vi "HMF_Factorial.vi"() -> ()   [LabVIEW 2015]
uses:
  <vilib>/Platform/TimedLoop/XDataNode/timing_clust.ctl
  <vilib>/Platform/TimedLoop/XDataNode/nitl_modes.ctl
  <vilib>/Platform/TimedLoop/XDataNode/wakeup.ctl
  <vilib>/DAQmx/read.llb/DAQmx Read (Analog DBL 1Chan 1Samp).vi
  <vilib>/DAQmx/read.llb/DAQmx Read (Analog 1D DBL NChan 1Samp).vi
  <vilib>/DAQmx/create/channels.llb/DAQmx Create Channel (AI-Voltage-Basic).vi
  <vilib>/Enthought/Python Integration Toolkit/api/Unpack Double.vi
  <vilib>/DAQmx/miscellaneous.llb/DAQmx Fill In Error Info.vi
  <vilib>/Platform/TimedLoop/XDataNode/XDataNode.xnode
  Program Files/neMESYS_SDK/neMESYS LabVIEW Kit/neMESYS LabVIEW Integration Kit.lvlib
  <vilib>/Platform/TimedLoop/XDataNode/XDNodeRunTimeDep.lvlib
  Conor/Temp CN7500/Omega CN7500/Omega CN7500.lvlib
  <vilib>/Enthought/Python Integration Toolkit/Python Integration Toolkit.lvlib
panel:
  in  "Temp  Limit OFF or ON":bool
  out "syringe limit empty":bool
  out "Pressure limit reached":bool
  out "Temp limit reached":bool
  in  "NaOH in 3 or NaOH in 2":bool
  out "N2 Cal 4":dbl
  out "N2 Cal 3":dbl
  out "N2 Cal 2":dbl
  out "O2 Cal 1":dbl
  out "C FDCA 8":dbl
  out "C FFCA 8":dbl
  out "C FDCA 7":dbl
  out "C FFCA 7":dbl
  out "C FDCA 6":dbl
  out "C FFCA 6":dbl
  out "C FDCA 5":dbl
  out "C FFCA 5":dbl
  out "C FDCA 4":dbl
  out "C FFCA 4":dbl
  out "C FDCA 3":dbl
  out "C FFCA 3":dbl
  out "C FDCA 2":dbl
  out "C FFCA 2":dbl
  out "C FDCA 1":dbl
  out "C FFCA 1":dbl
  out "O2 frac 8":dbl
  in  "O2 frac 8":dbl
  out "O2 frac 7":dbl
  in  "O2 frac 7":dbl
  out "O2 frac 6":dbl
  in  "O2 frac 6":dbl
  out "O2 frac 5":dbl
  in  "O2 frac 5":dbl
  out "O2 frac 4":dbl
  in  "O2 frac 4":dbl
  out "O2 frac 3":dbl
  in  "O2 frac3":dbl
  out "O2 frac 2":dbl
  out "O2 frac 1":dbl
  in  "O2 frac 2":dbl
  in  "O2 frac 1":dbl
  in  "O2 frac 0":dbl
  in  "Total Gas Flow Rate":dbl
  in  "Back Pressure Bar Abs":dbl
  in  "Test Gas Communication":bool
  in  "Read Set Points":bool
  in  "Change New Set Points":bool
  out "Text Read From Clipboard 5":string
  out "Read error out 5":errorcluster
  out "Write Set Point Status 2":string
  out "Error Out 5":i32
  out "Write error out 5":errorcluster
  out "Text Read From Clipboard 4":string
  out "Read error out 4":errorcluster
  out "Write Set Point Status":string
  out "Error Out 4":i32
  out "Write error out 4":errorcluster
  in  "Set Point 1 (NmL/min)":dbl
  in  "Set Point 2 (NmL/min)":dbl
  in  "Set Point 3 (NmL/min)":dbl
  out "Flow Span of All Controlers (NmL/min)":dbl
  in  "Set Point 4 (NmL/min)":dbl
  out "Set Point Function":string
  out "Text Read From Clipboard 3":string
  out "Read error out 3":errorcluster
  out "Read Set Point Status":string
  out "Error Out 3":i32
  out "Write error out 3":errorcluster
  out "Text Read From Clipboard":string
  out "Read error out":errorcluster
  out "Test Status":string
  out "Error Out":i32
  out "Write error out":errorcluster
  out "Text Read From Clipboard 2":string
  out "Read error out 2":errorcluster
  out "Read Flow Status":string
  out "Gas Flow 1 NmL/min":dbl
  out "Gas Flow 2 NmL/min":dbl
  out "Gas Flow 3 NmL/min":dbl
  out "Gas Flow 4 NmL/min":dbl
  out "Gas Flow rate":dynamicdata(graph)
  out "First waste string":string
  out "Rest of string 1":string
  out "First Number":string
  out "Rest of string 2":string
  out "Second Number 2":string
  out "Rest of string 3":string
  out "Third Number 3":string
  out "Rest of string 4":string
  out "Fourth Number 3":string
  out "Rest of string 5":string
  out "Error Out 2":i32
  out "Write error out 2":errorcluster
  out "Nitrogen Pressure (barg)":dbl
  out "Reactor Gas Back Pressure (barg)":dbl
  out "Nitrogen Gas  Pressure (barg)":dbl
  out "Slope 4":dbl
  out "Slope 3":dbl
  out "Slope 2":dbl
  out "Intercept 4":dbl
  out "Intercept  3":dbl
  out "Intercept 2":dbl
  out "Intercept 1":dbl
  out "Slope 1":dbl
  in  "2 Syringes or 4 Syringes":bool
  in  "Conc NaOH in Syringe":dbl
  in  "Cat Mass mg":dbl
  out "Exp 2":bool
  out "C HFCA 1":dbl
  out "C HMF 1":dbl
  out "Exp 9":bool
  out "Liquid Inlet Pressure (bar g)":dbl
  in  "Liquid P sensor Terminal Configuration":i32(ring)=-1 items=["default"=-1, "RSE"=10083, "NRSE"=10078, "Differential"=10106, "Pseudodifferential"=12529]
  in  "Liquid P sensor Physical Channel":tag="Dev1/ai0"
  in  "Temp 2":dbl
  in  "Conc 2":dbl
  in  "Flow 2":dbl
  out "Exp 8":bool
  out "Exp 7":bool
  out "Exp 6":bool
  out "Exp 5":bool
  out "Exp 4":bool
  out "Exp 3":bool
  out "Exp 1":bool
  out "Exp 0":bool
  out "C HMF 8":dbl
  out "C HFCA 8":dbl
  in  "Flow 8":dbl
  in  "Conc 8":dbl
  in  "Temp 8":dbl
  out "Temp 8":dbl
  out "Flow 8":dbl
  out "Conc 8":dbl
  out "C HMF 7":dbl
  out "C HFCA 7":dbl
  in  "Flow 7":dbl
  in  "Conc 7":dbl
  in  "Temp 7":dbl
  out "Temp 7":dbl
  out "Flow 7":dbl
  out "Conc 7":dbl
  out "C HMF 6":dbl
  out "C HFCA 6":dbl
  in  "Flow 6":dbl
  in  "Conc 6":dbl
  in  "Temp 6":dbl
  out "Temp 6":dbl
  out "Flow 6":dbl
  out "Conc 6":dbl
  out "C HMF 5":dbl
  out "C HFCA 5":dbl
  in  "Flow 5":dbl
  in  "Conc 5":dbl
  in  "Temp 5":dbl
  out "Temp 5":dbl
  out "Flow 5":dbl
  out "Conc 5":dbl
  out "C HMF 4":dbl
  out "C HFCA 4":dbl
  out "Conc 1":dbl
  out "Flow 1":dbl
  out "Temp 1":dbl
  out "Conc 2":dbl
  out "Flow 2":dbl
  out "Temp 2":dbl
  in  "Flow 4":dbl
  in  "Conc 4":dbl
  in  "Temp 4":dbl
  out "Temp 4":dbl
  out "Flow 4":dbl
  out "Conc 4":dbl
  out "C HMF 3":dbl
  out "C HFCA 3":dbl
  out "Conc 3":dbl
  out "Flow 3":dbl
  out "Temp 3":dbl
  out "C HMF 2":dbl
  out "C HFCA 2":dbl
  in  "Temp 3":dbl
  in  "Conc 3":dbl
  in  "Flow 3":dbl
  in  "Result file name -  needs extension RecordHMF.xlsx":string
  in  "HPLC file Name -doesnt need extension":string
  out "Desired Conc Not Possible":bool
  in  "Safety or Emergency Syringe Control":bool
  out "Feed Concentration if 2 syringe (M)":dbl
  out "Total Flowrate (uL/min)":dbl
  out "Oxygen Gas Pressure (barg)":dbl
  in  "Shut down in empty?\nLeft off, right on":bool
  out "Safety Shut Down Pressure (barg)":dbl
  out "Safety Shut Down Temp":dbl
  out "Actual Temp (oC)":dbl
  out "Temperature":dynamicdata(graph)
  out "Temp Set Point (oC)":dbl
  in  "Temp 1":dbl
  in  "Temp 0":dbl
  in  "Update Temperature Set Point":bool
  in  "Automated Experiments or Direct Control":bool
  in  "Set Point (oC)":dbl
  out "loop ind":dbl
  in  "Stop everything":bool
  in  "Skip Exp":bool
  in  "Minutes between Exp":dbl min=0.0 step=0.05
  in  "Refill 4":bool
  in  "Refill 3":bool
  in  "Refill 2":bool
  in  "Refill 1":bool
  in  "Empty 4":bool
  in  "Empty 3":bool
  in  "Empty 2":bool
  in  "Empty 1":bool
  in  "Calibrate 4":bool
  in  "Calibrate 3":bool
  in  "Calibrate 2":bool
  in  "Calibrate 1":bool
  in  "Stop Dose 4":bool
  in  "Stop Dose 3":bool
  in  "Stop Dose 2":bool
  in  "Stop Dose 1":bool
  in  "Flow 1":dbl
  in  "Conc 1":dbl
  in  "Flow 0":dbl
  in  "Conc 0  (M)":dbl
  in  "Generate Flow":bool
  in  "Set Flowrate 1":dbl
  in  "Set Flowrate 2":dbl
  in  "Set Flowrate 3":dbl
  in  "Set Flowrate 4":dbl
  out "High Conc":dbl min=0.0 max=2.0
  out "Low Conc":dbl min=0.0 max=2.0
  out "Syringe Level 4":dbl(slide) scale=0.0..5500.0
  out "Syringe Level 3":dbl(slide) scale=0.0..5500.0
  out "Syringe Level 2":dbl(slide) scale=0.0..5500.0
  out "Syringe Level 1":dbl(slide) scale=0.0..5500.0
  out "Flowrate 4 NaOH":dbl
  out "Flowrate 3 NaOH":dbl
  out "Flowrate 2 NaOH or HMF":dbl
  out "Flowrate 1 HMF":dbl
  # "Current Conditions"
  # "Pre Planned Experiments"
  # "Conducted Experiments Set Points"
  # "example file name to show correct format is..."
  # "HMF_HPLC"
  # "(uL/min)"
  # "Coerced to nearest possible"
  # "Factorial Only"
  # "Experimental Info"
  # "Direct Control"
  # "Emergency Syringe Control Below"
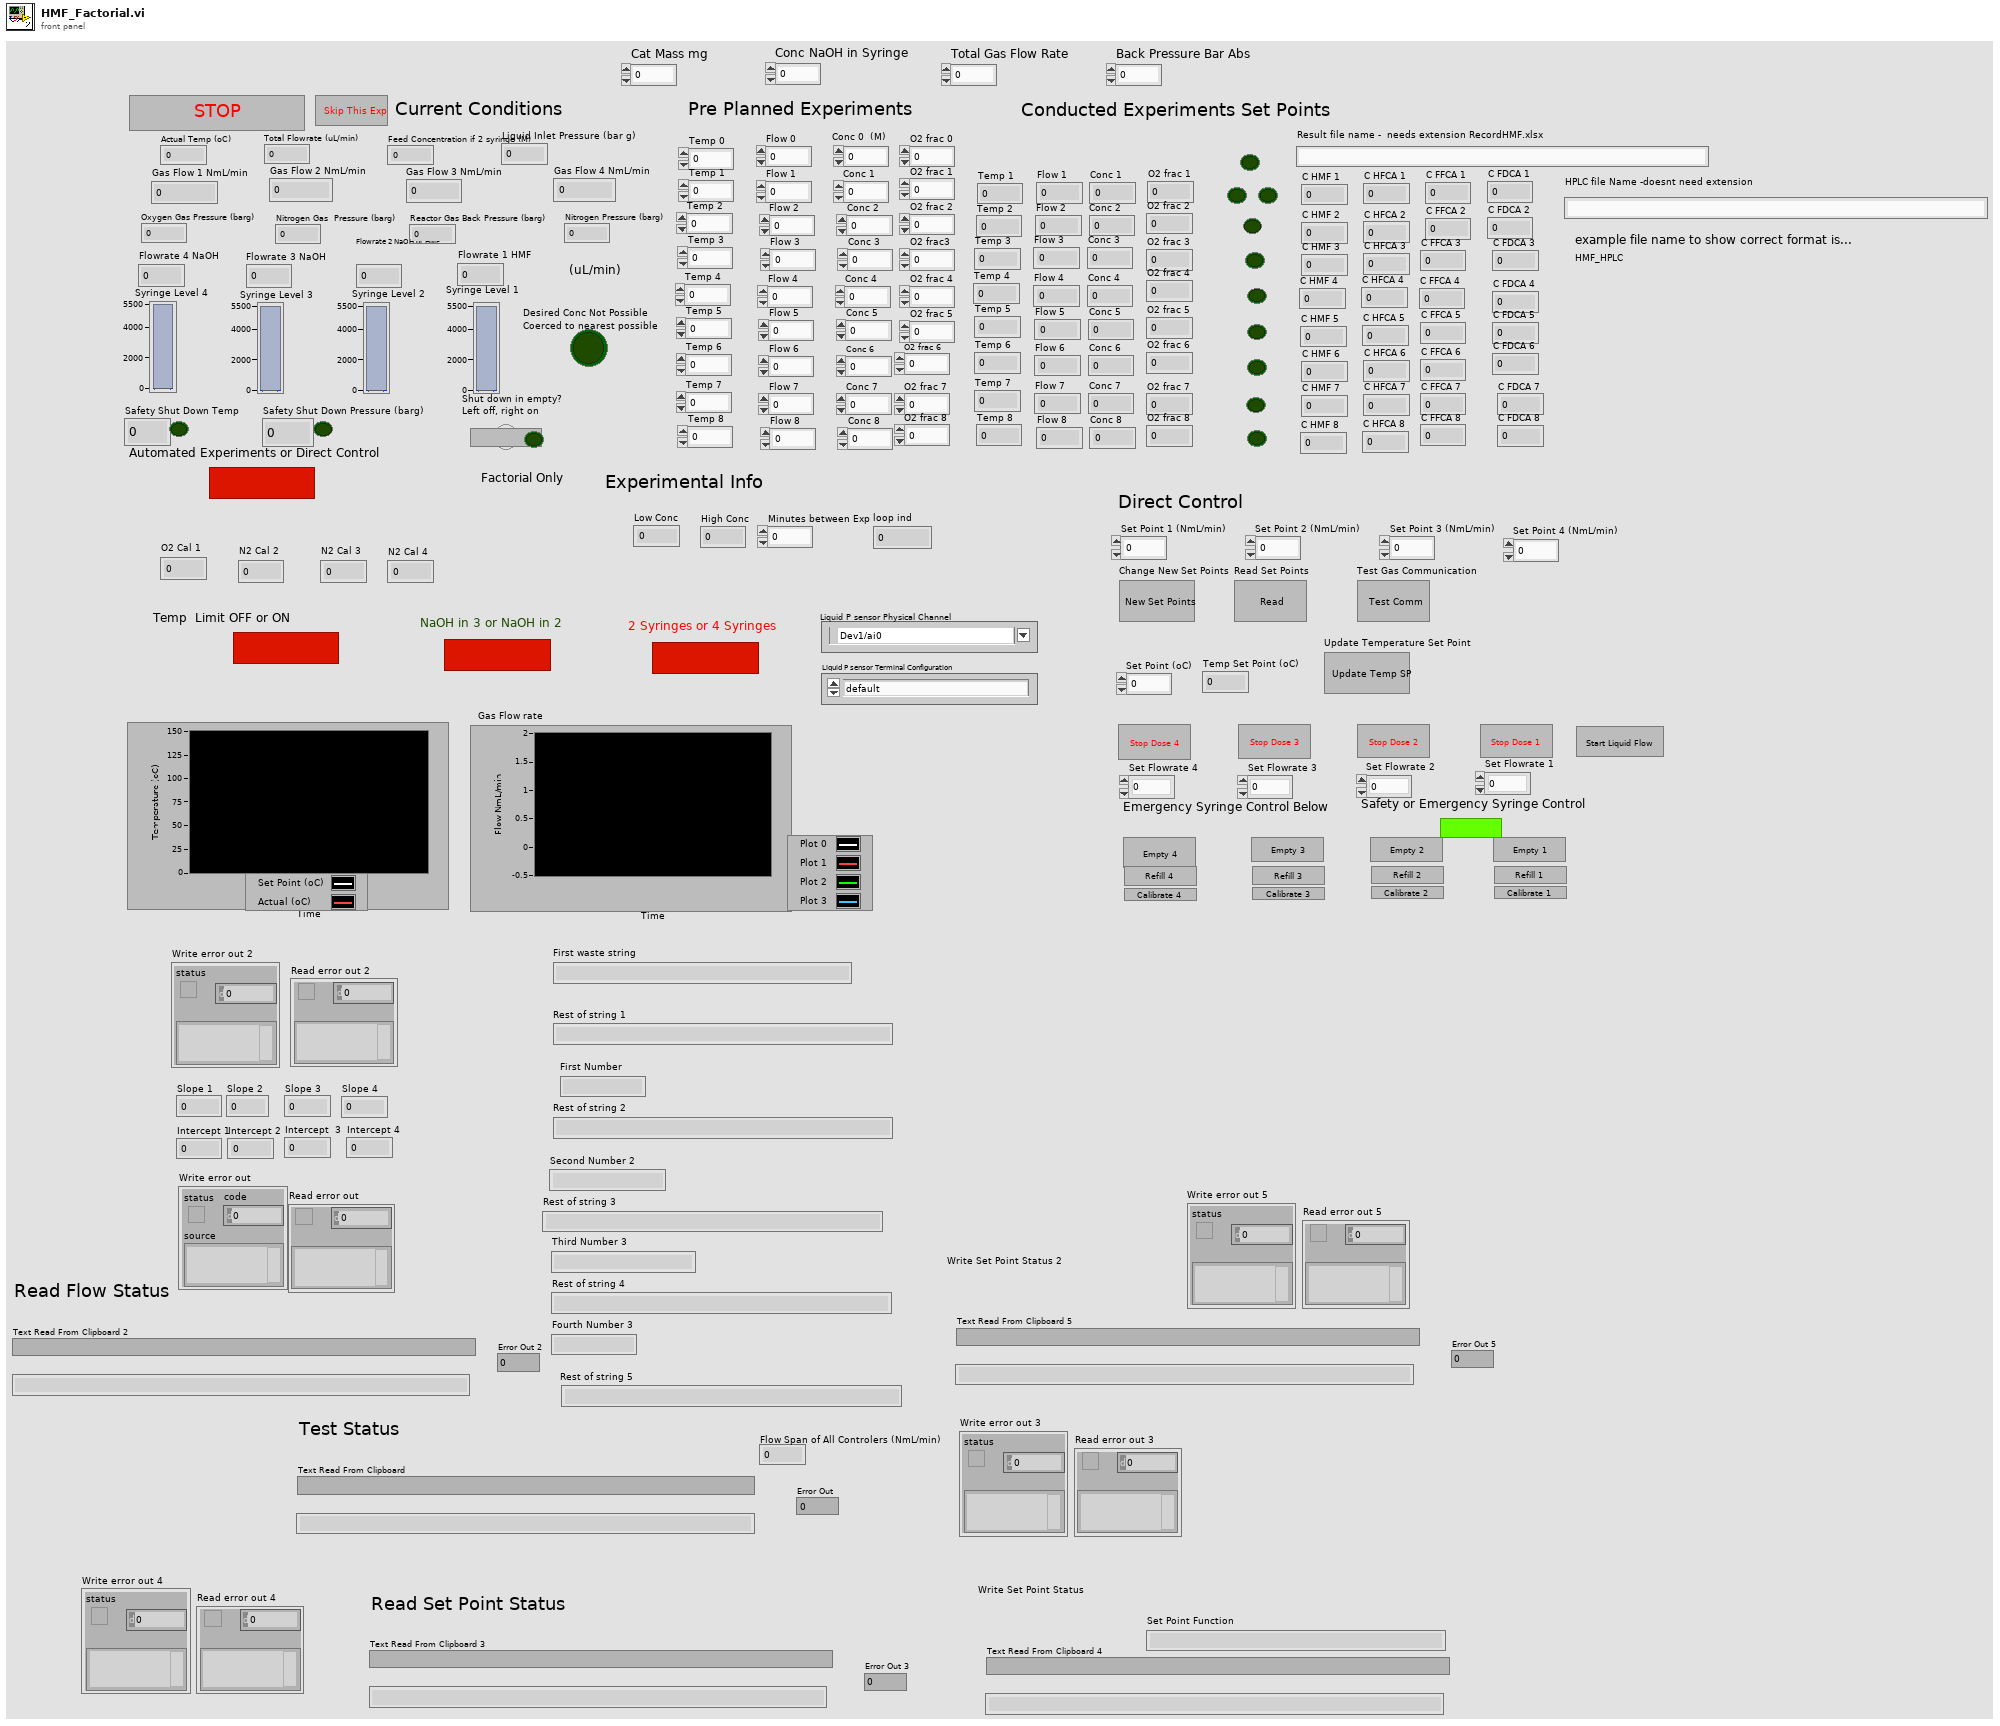
[diagram p1: front panel]
types:
  T1 = typedef "XDNodeRunTimeDep.lvlib/timing_clust.ctl" = cluster{"Expected End [f-1]":u64, "Actual End [f-1]":u64, "Finished Late? [f-1]":bool, "Expected End [i-1]":u64, "Actual End [i-1]":u64, "Finished Late? [i-1]":bool, "Expected Start [i]":u64, "Actual Start [i]":u64, "Expected Start [f]":u64, "Actual Start [f]":u64, "Source Name":string, "Structure Name":string, "Period":i64, "Deadline":i64, "Offset":i64, "Start":i64, "Priority":i32, "Timeout":i32, "Mode":T2, "Wakeup Reason":T3, "Error":errorcluster, "Source Type":string, "Secondary Source Type":string, "Global End Time":u64, "Global Start Time":u64, "Frame Duration":u64, "Iteration Duration":u64, "Assigned CPU":i32, "I/O Scan Engine Mode":u32}
  T2 = typedef "XDNodeRunTimeDep.lvlib/nitl_modes.ctl" = enum32{"No Change", "Process missed periods, maintain original phase", "Discard missed periods, maintain original phase", "Process missed periods, ignore original phase", "Discard missed periods, ignore original phase"}
  T3 = typedef "XDNodeRunTimeDep.lvlib/wakeup.ctl" = enum32{"Normal", "Aborted", "Asynchronous wakeup", "Timing source error", "Timed loop error", "Timeout"}
  T4 = typedef "Python Integration Toolkit.lvlib/Session ID.ctl" = u64
  T5 = typedef "Python Integration Toolkit.lvlib/Python Objects.ctl" = variant
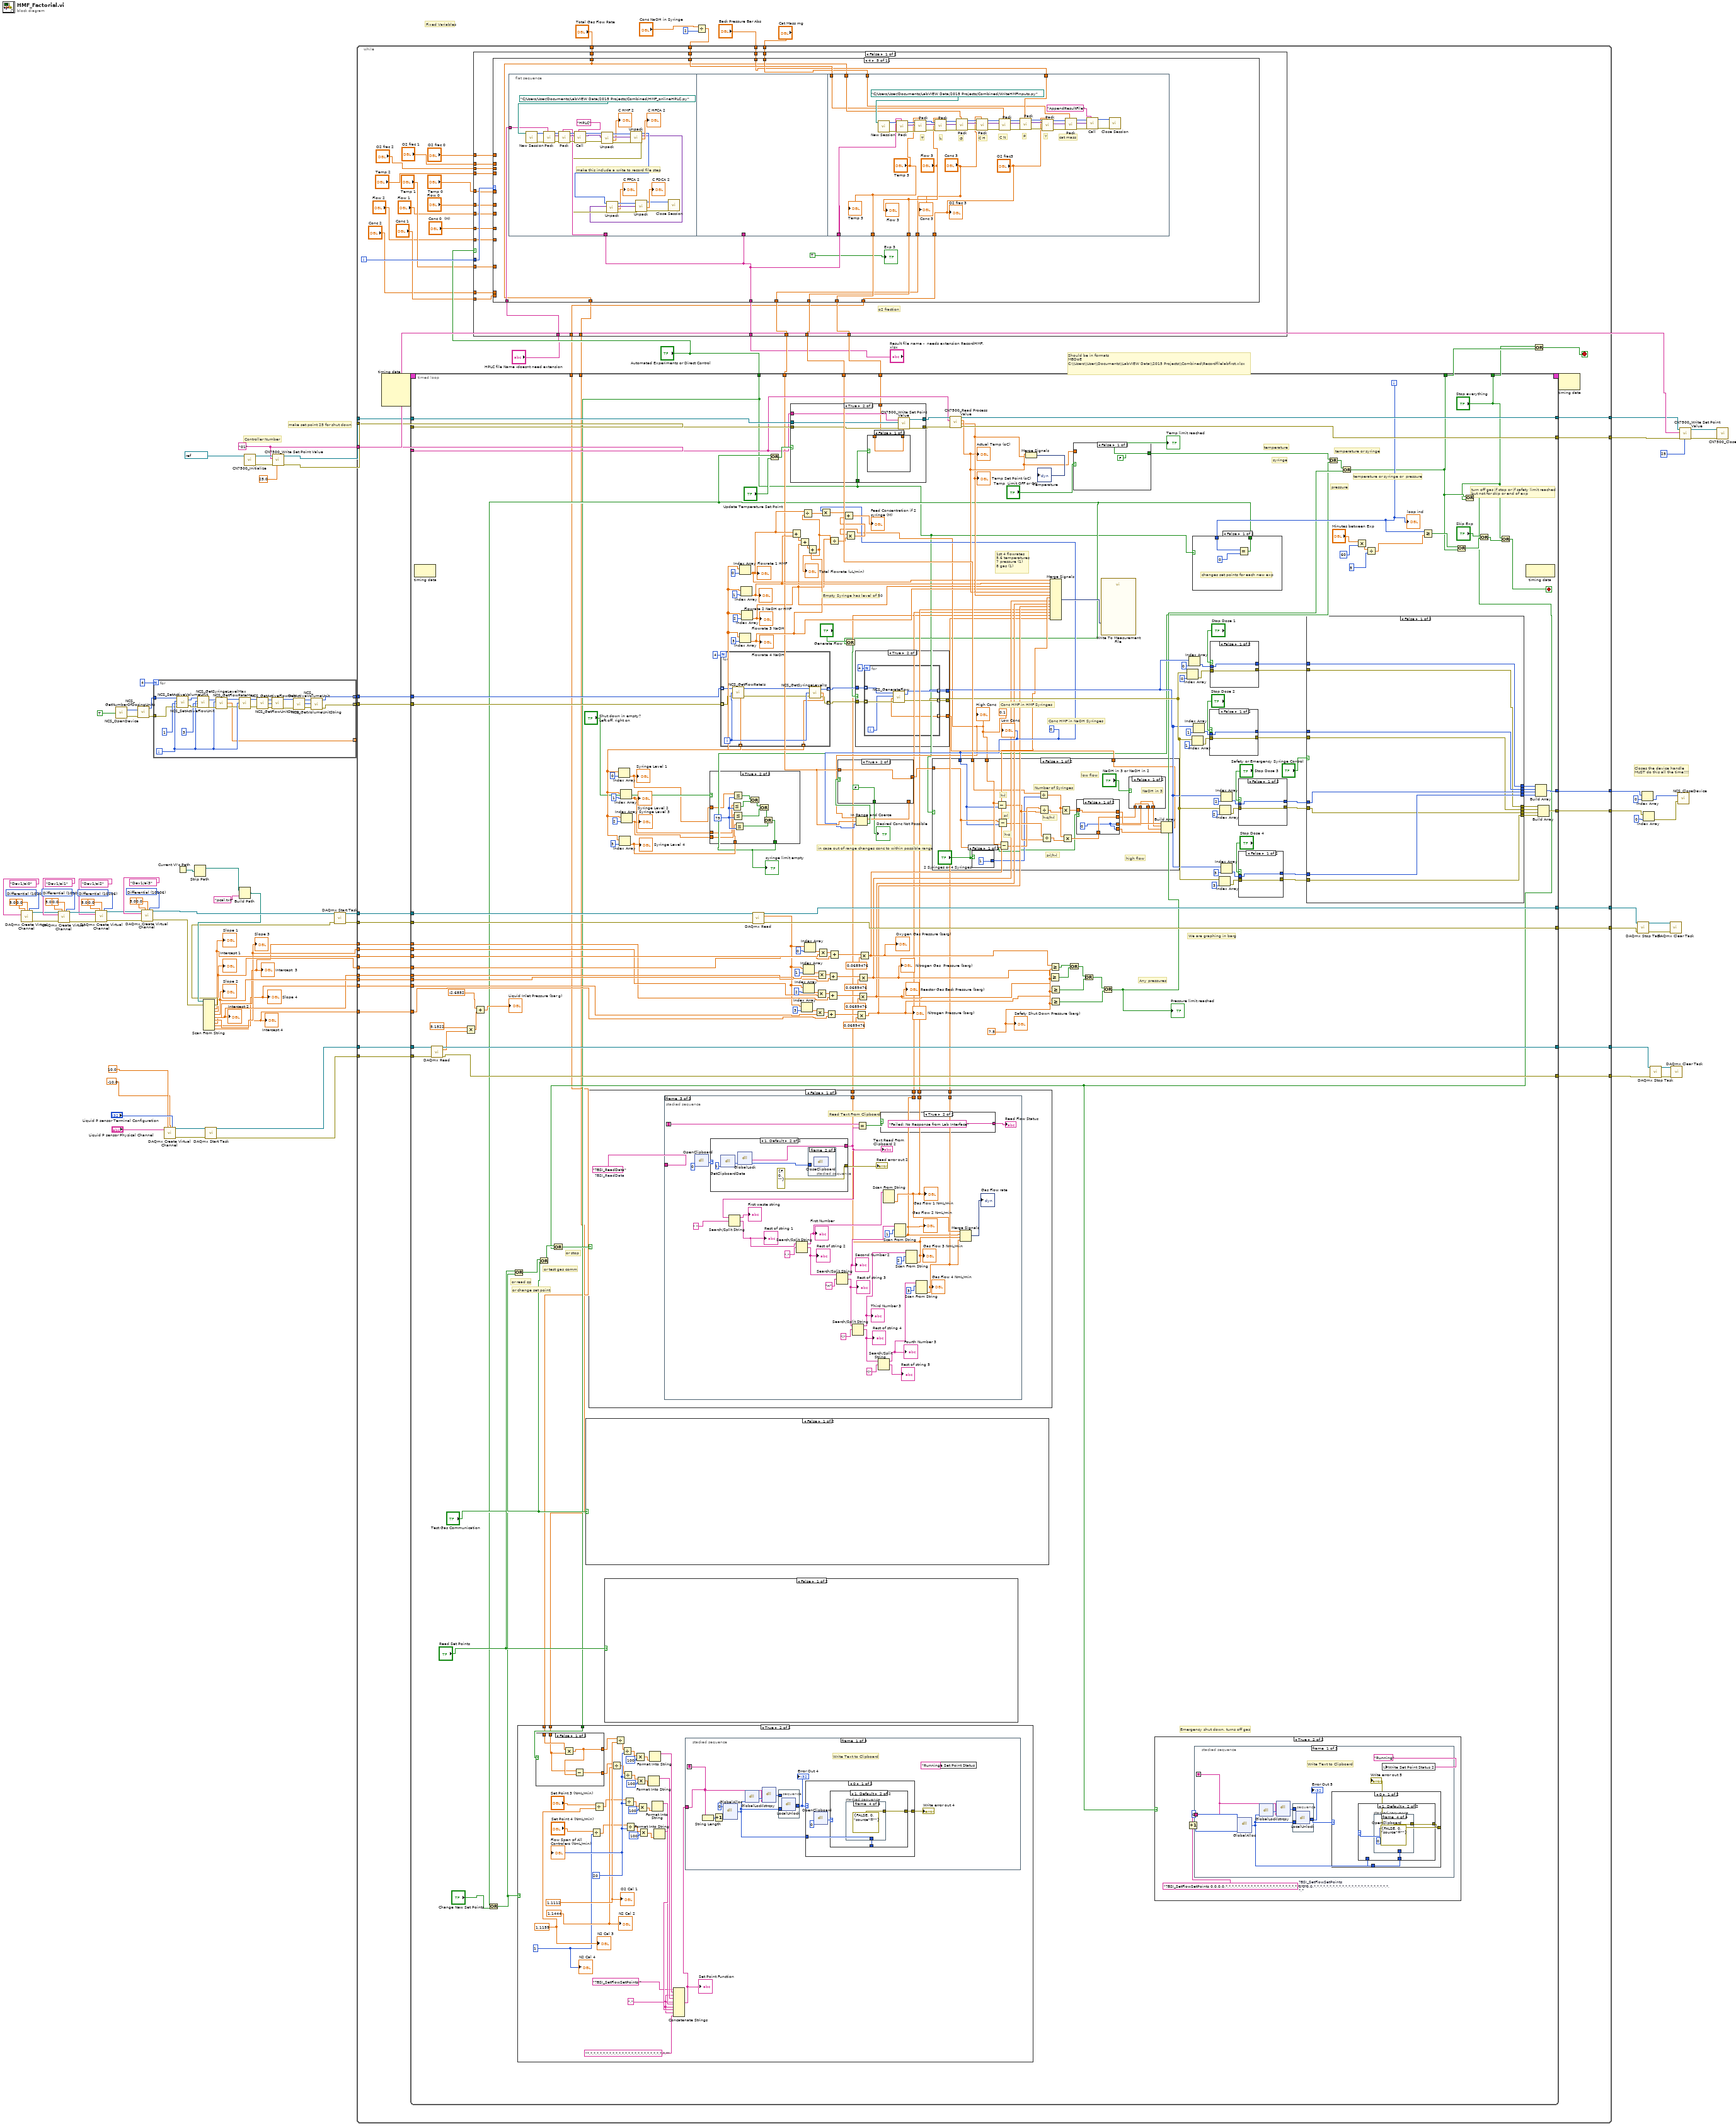
[diagram p0: block diagram]
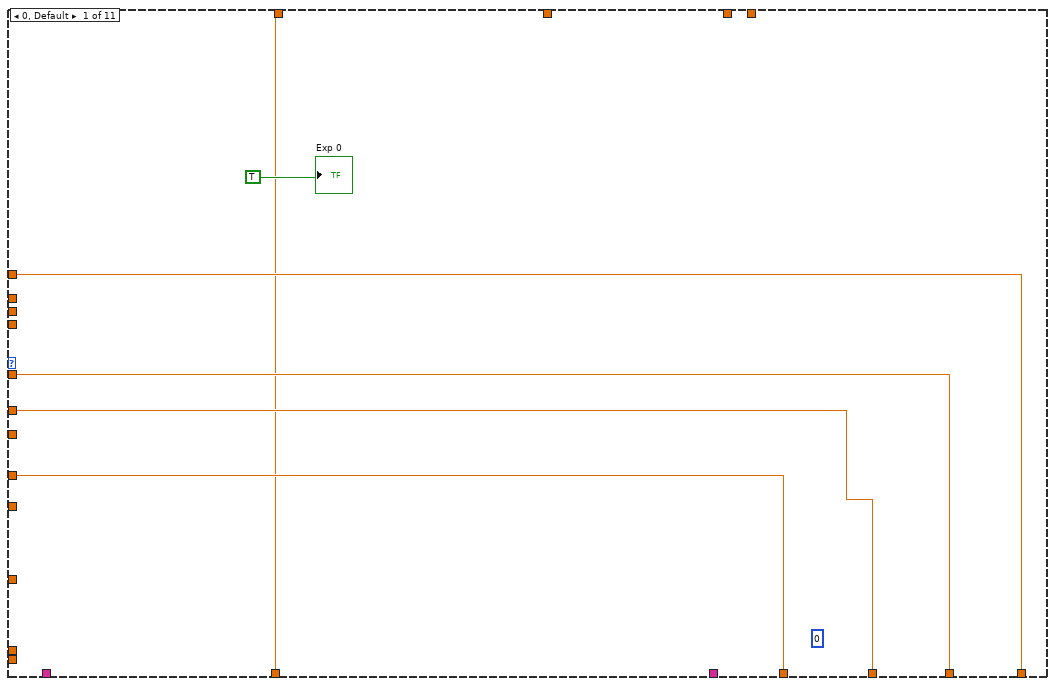
[diagram p2: hidden frame]
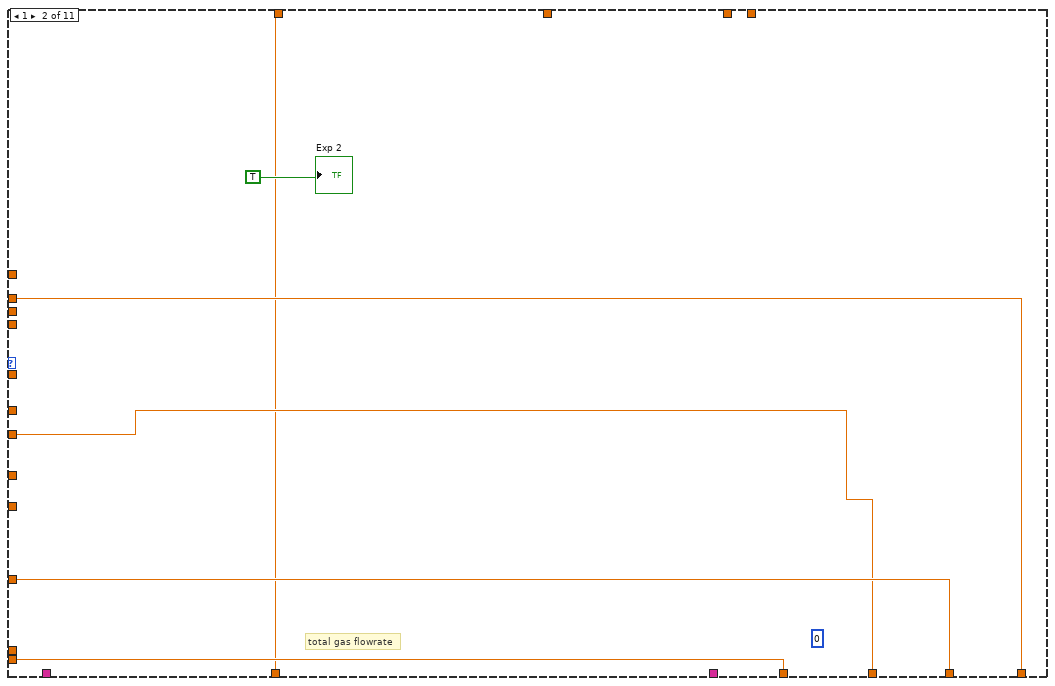
[diagram p3: hidden frame]
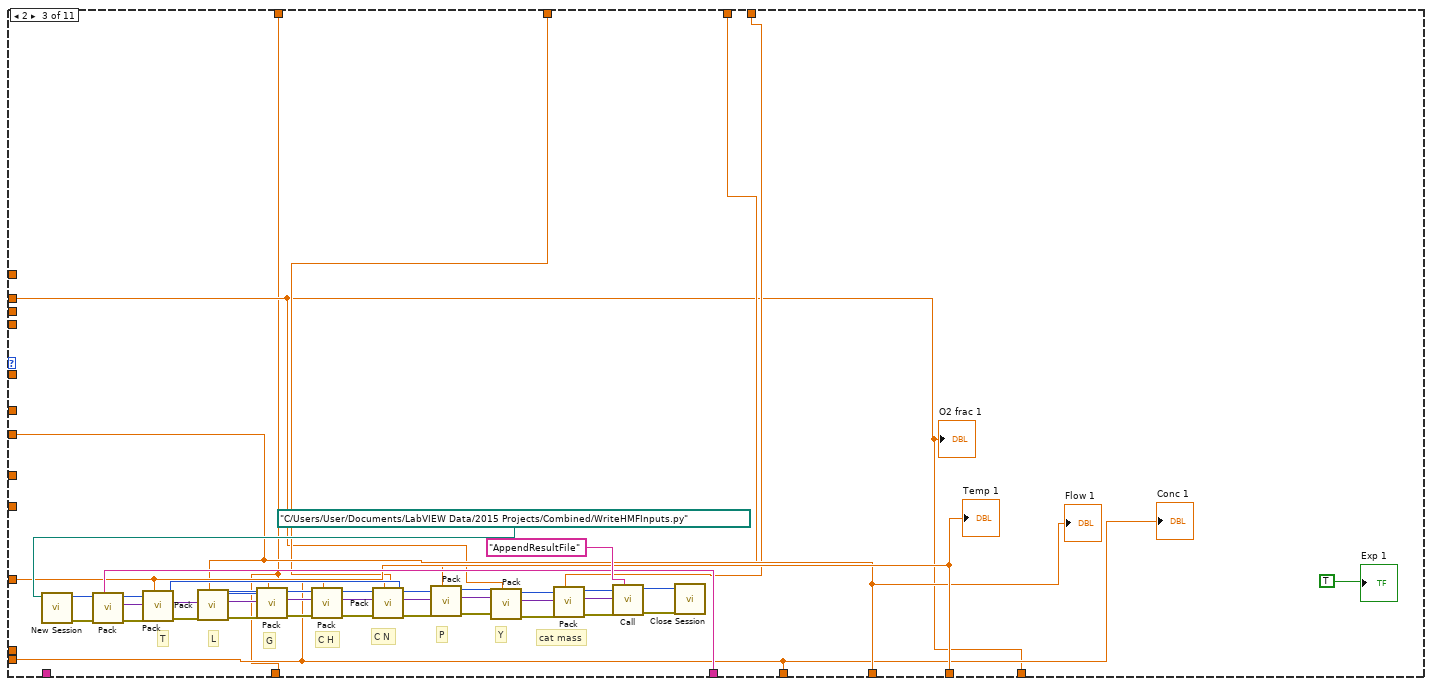
[diagram p4: hidden frame]
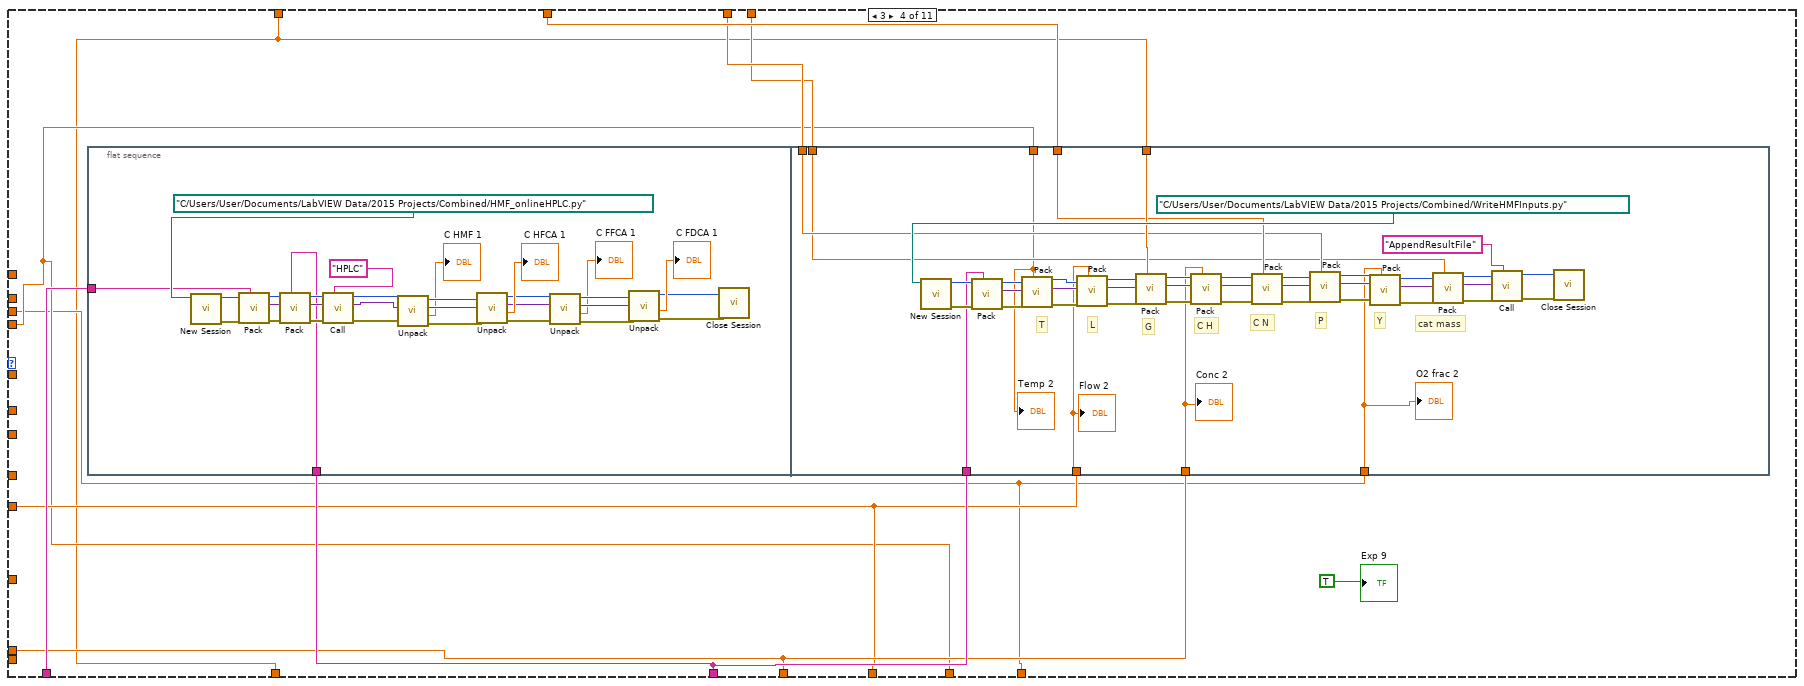
[diagram p5: hidden frame]
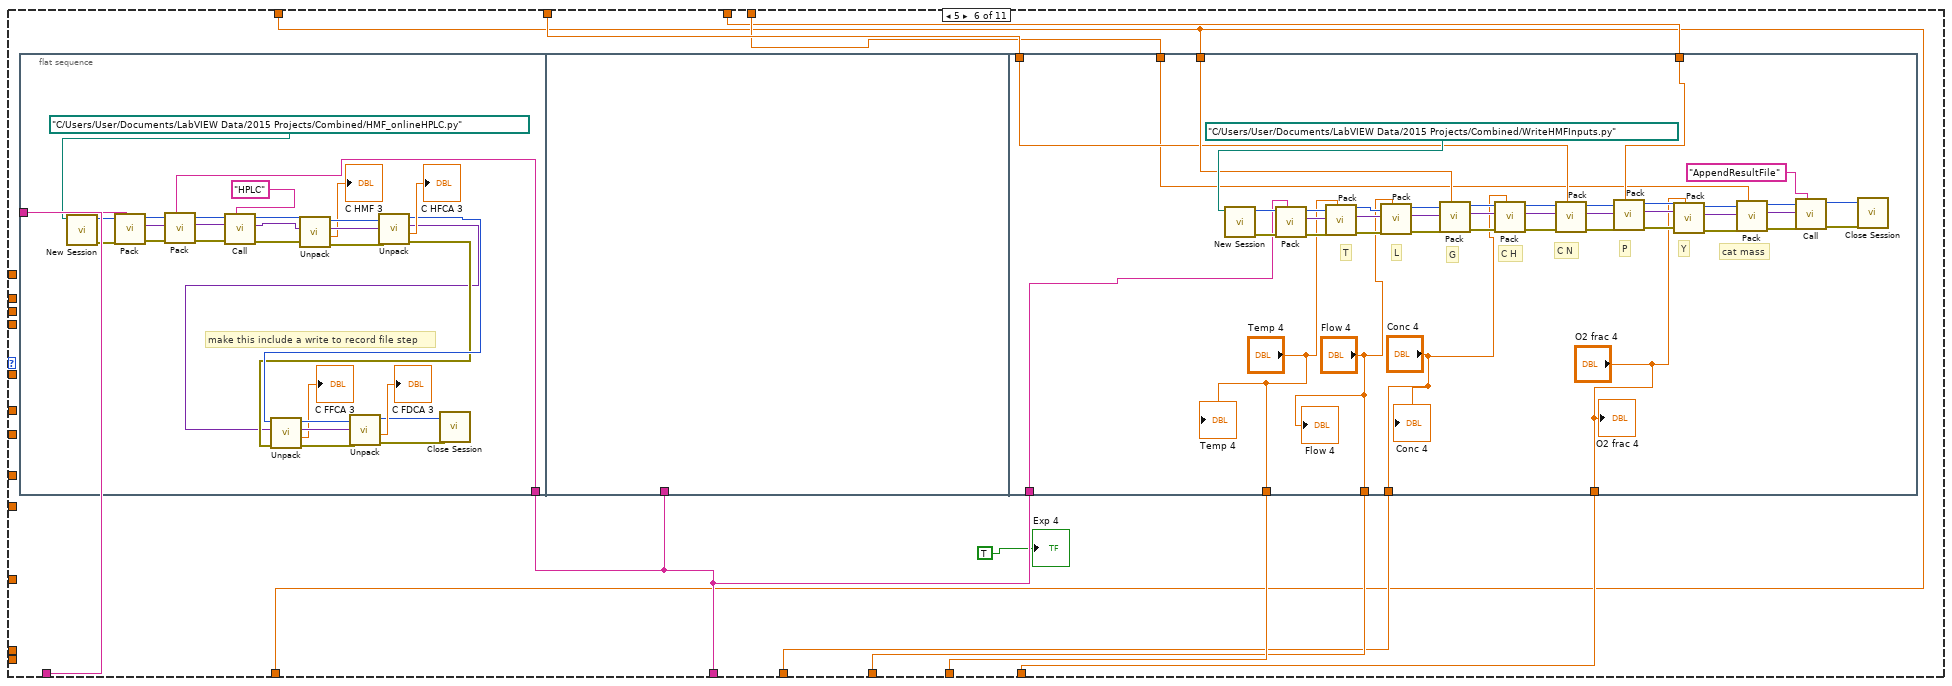
[diagram p6: hidden frame]
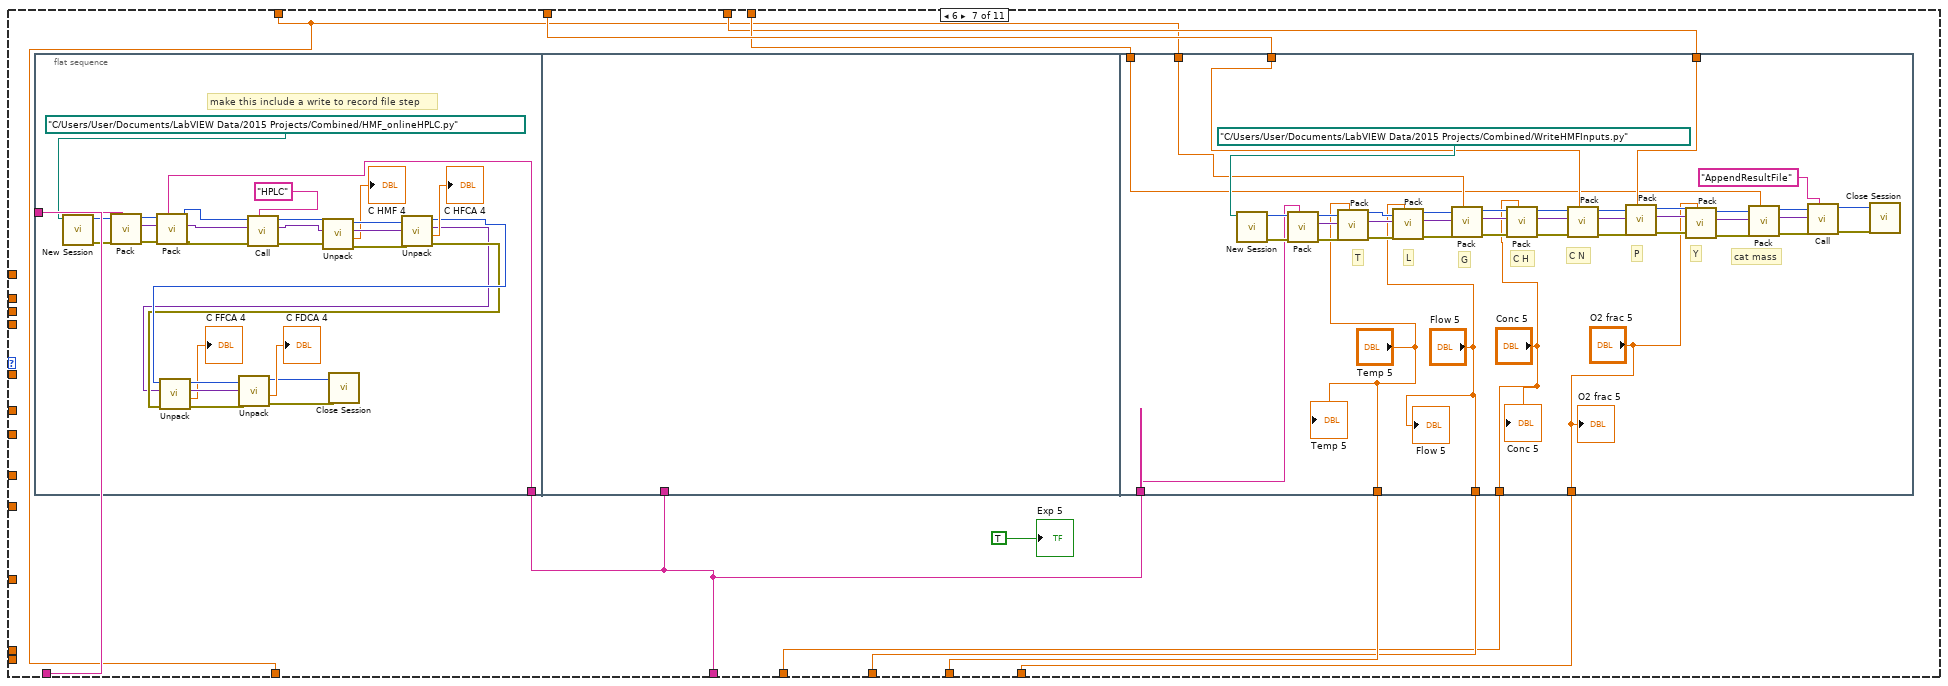
[diagram p7: hidden frame]
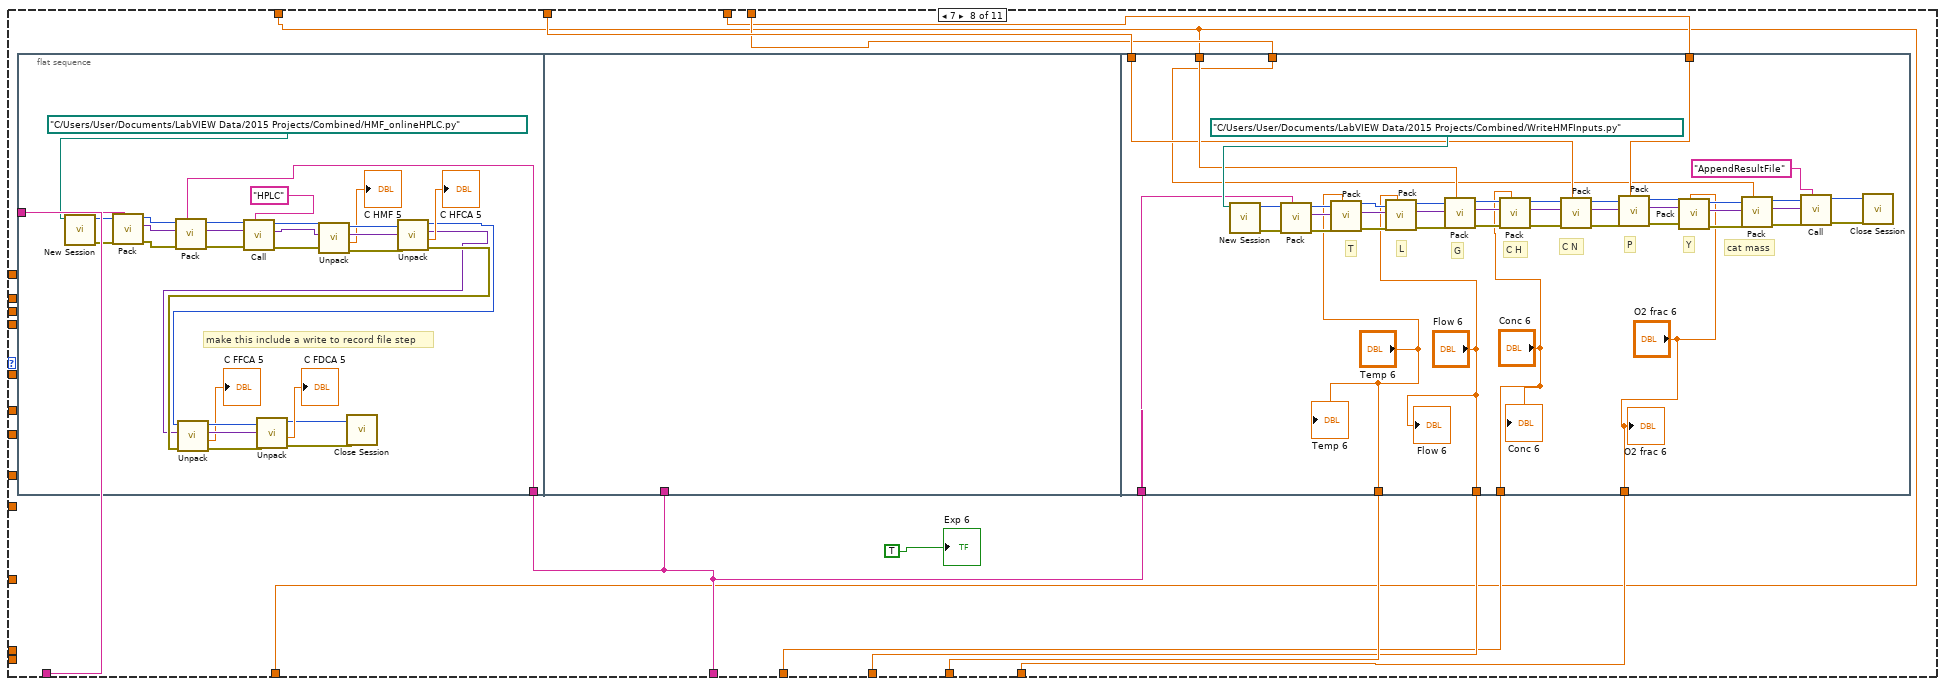
[diagram p8: hidden frame]
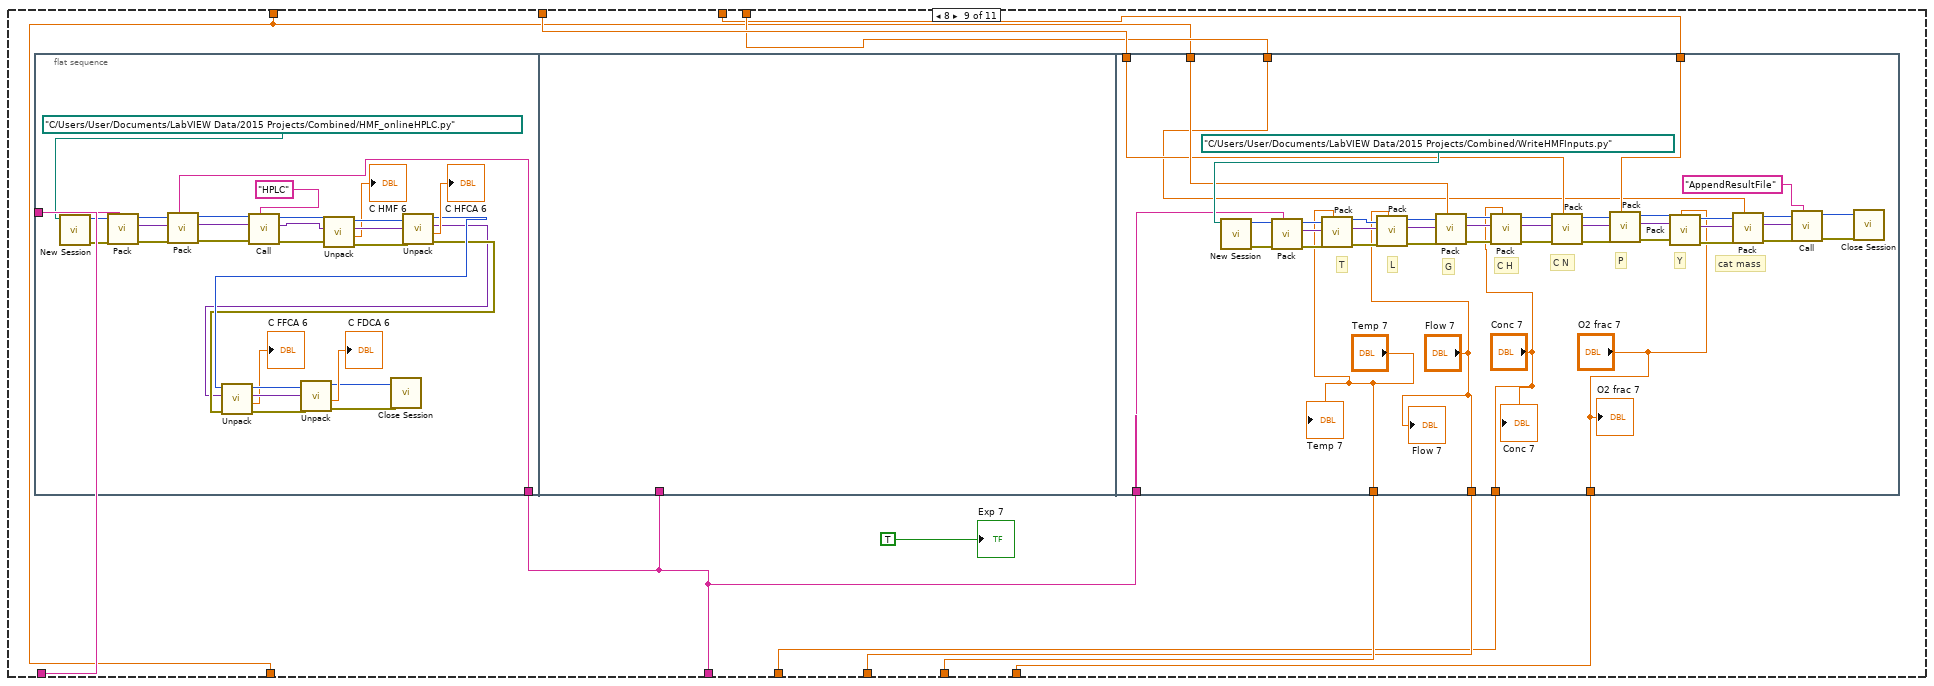
[diagram p9: hidden frame]
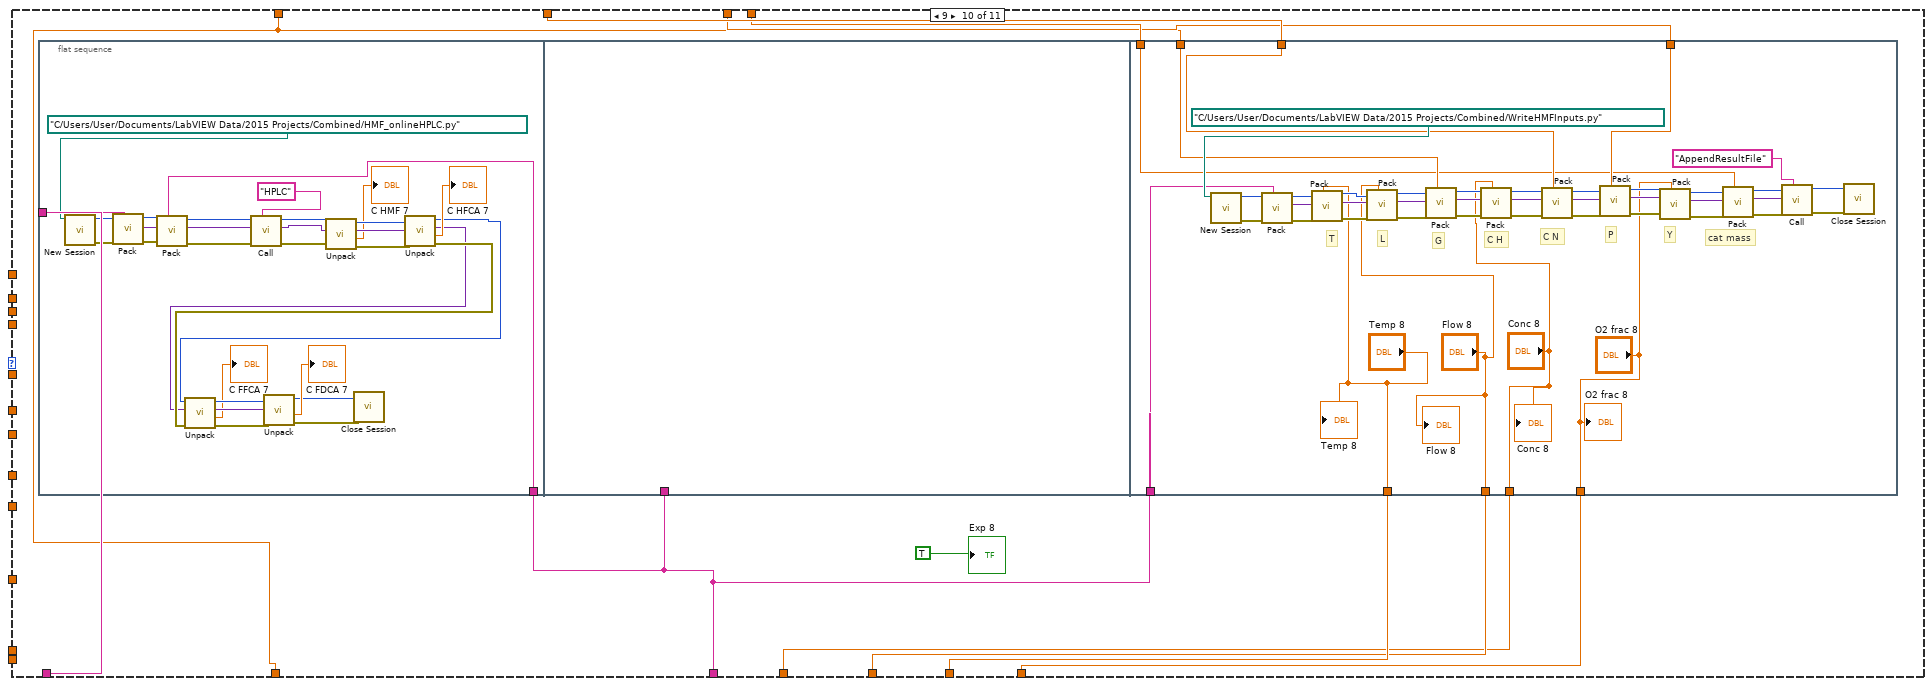
[diagram p10: hidden frame]
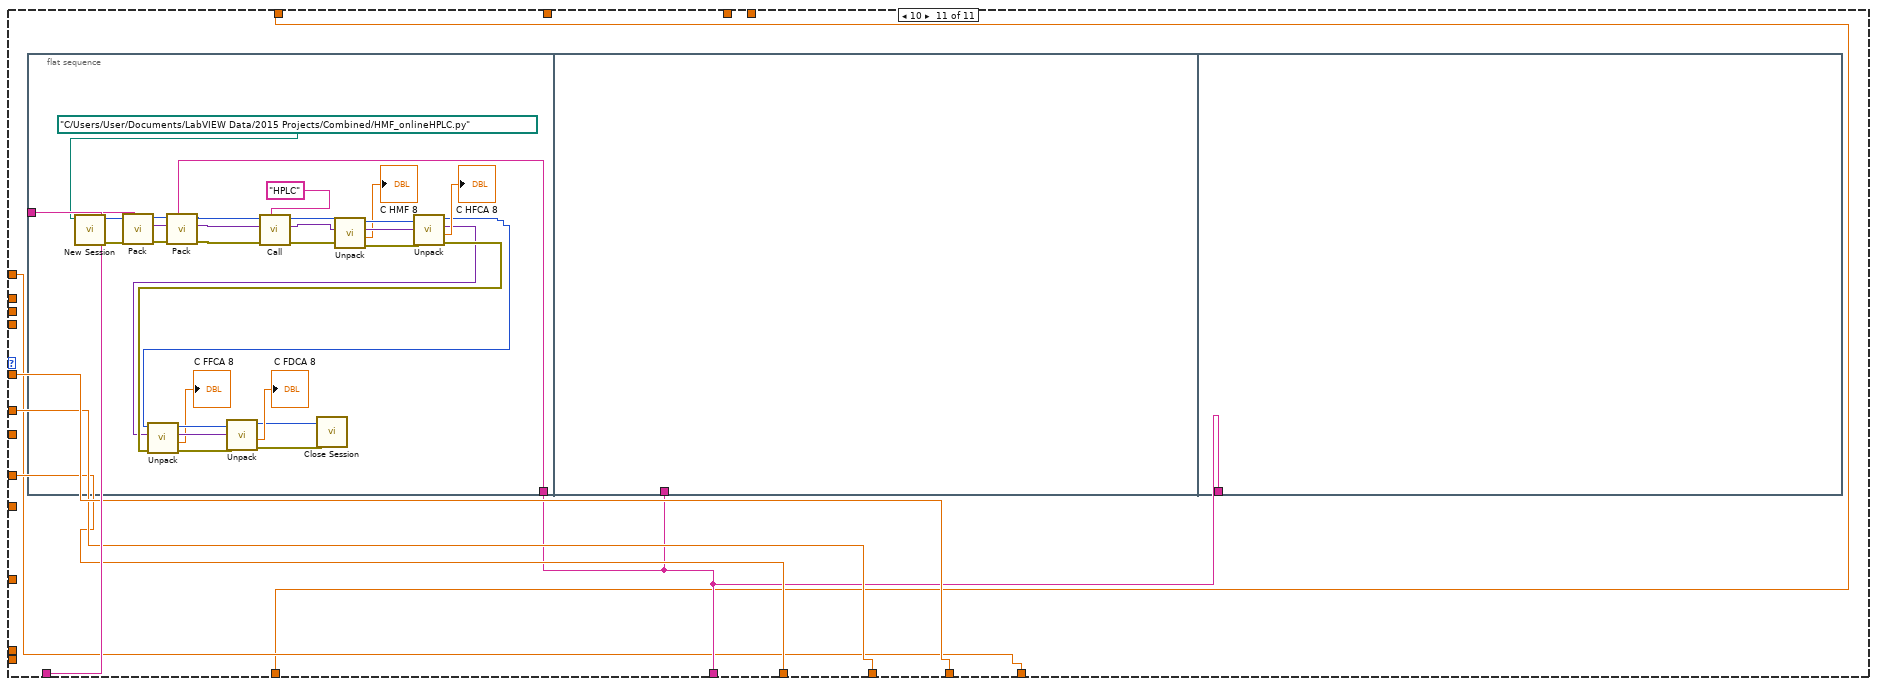
[diagram p11: hidden frame]
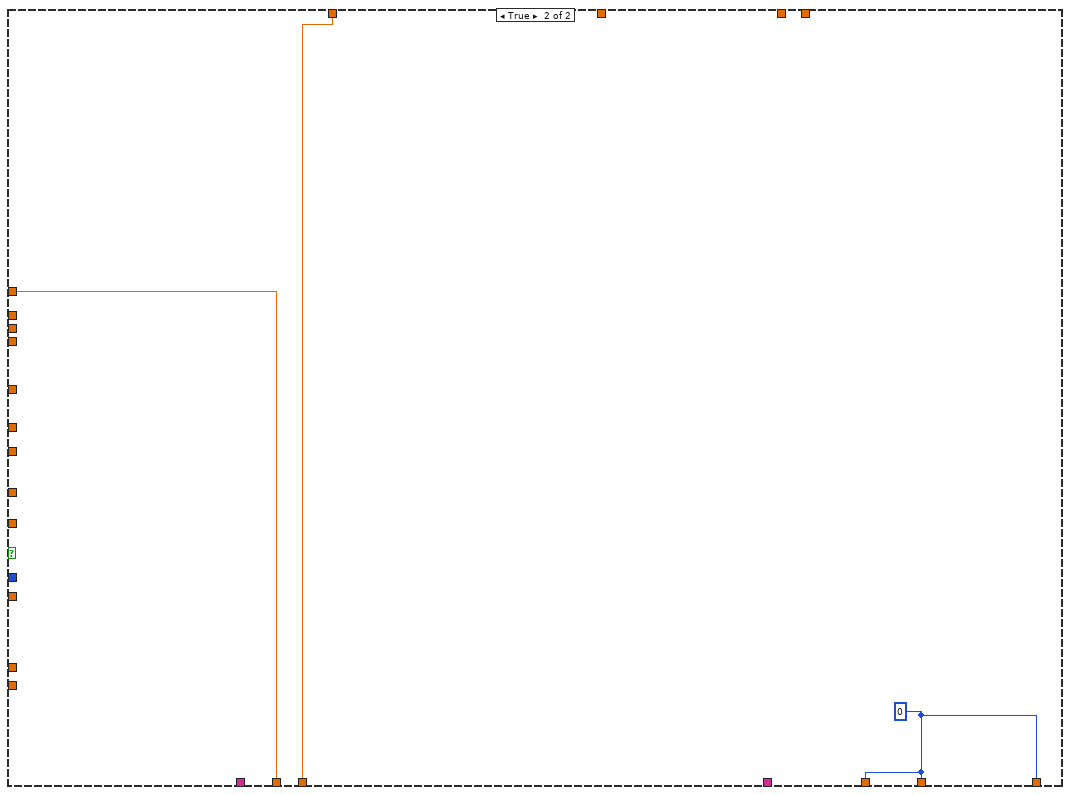
[diagram p12: hidden frame]
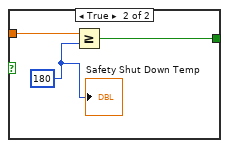
[diagram p13: hidden frame]
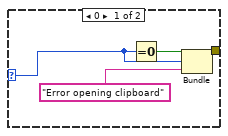
[diagram p15: hidden frame]
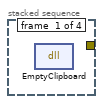
[diagram p16: hidden frame]
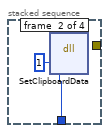
[diagram p17: hidden frame]
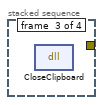
[diagram p18: hidden frame]
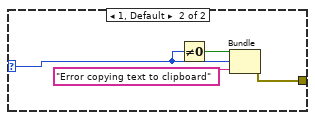
[diagram p19: hidden frame]
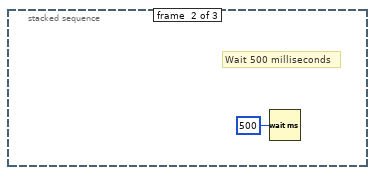
[diagram p20: hidden frame]
diagram:
  w22 = 10106 items=["default"=-1, "RSE"=10083, "NRSE"=10078, "Differential"=10106, "Pseudodifferential"=12529] ("input terminal configuration")
  w30 = 10106 items=["default"=-1, "RSE"=10083, "NRSE"=10078, "Differential"=10106, "Pseudodifferential"=12529] ("input terminal configuration")
  w17 = 10106 items=["default"=-1, "RSE"=10083, "NRSE"=10078, "Differential"=10106, "Pseudodifferential"=12529] ("input terminal configuration")
  w59 = 10106 items=["default"=-1, "RSE"=10083, "NRSE"=10078, "Differential"=10106, "Pseudodifferential"=12529] ("input terminal configuration")
  w66 = "01" ("Controller Number")
  # "Fixed Variables"
  # "make set point 25 for shut down"
  # "Controller Number"
  # "Closes the device handle \nMUST do this all the time!!!!"
  n1 = call-poly <vilib>:"DAQmx Create Virtual Channel.vi"("maximum value"=5.0, "minimum value"=0.0, "input terminal configuration"=w22, "physical channels"=tag "Dev1/ai0") -> ("task out"=w26:refnum<k21>, "error out"=w25:errorcluster)  [unwired: 10 in]
  n2 = call-poly <vilib>:"DAQmx Create Virtual Channel.vi"("task in"=w26, "maximum value"=5.0, "minimum value"=0.0, "input terminal configuration"=w30, "physical channels"=tag "Dev1/ai1", "error in"=w25) -> ("task out"=w28:refnum<k21>, "error out"=w27:errorcluster)  [unwired: 8 in]
  n3 = call-poly <vilib>:"DAQmx Create Virtual Channel.vi"("task in"=w28, "maximum value"=5.0, "minimum value"=0.0, "input terminal configuration"=w17, "physical channels"=tag "Dev1/ai2", "error in"=w27) -> ("task out"=w20:refnum<k21>, "error out"=w19:errorcluster)  [unwired: 8 in]
  n4 = call "NCS_OpenDevice.vi"("show status window"=TRUE) -> ("device handle"=w85:u32, "error out"=w84:errorcluster)
  n5 = call "NCS_GetNumberOfDosingUnits.vi"("device handle in"=w85, "error in (no error)"=w84) -> ("device handle out"=w82:u32, "error out"=w83:errorcluster)  [unwired: 1 out]
  n6 = call-poly <vilib>:"DAQmx Create Virtual Channel.vi"("task in"=w20, "maximum value"=5.0, "minimum value"=0.0, "input terminal configuration"=w59, "physical channels"=tag "Dev1/ai3", "error in"=w19) -> ("task out"=w48:refnum<k21>, "error out"=w16:errorcluster)  [unwired: 8 in]
  n7 = for {
    N: 4 -> [_]
    tunnel: [w91] -> w81 mode=indexing
    tunnel: [w90] -> w80 mode=indexing
    tunnel: [w104] -> _ mode=indexing
    tunnel: w83 -> [w89]
    tunnel: w82 -> [w88]
    i -> [w107]
    n8 = call "NCS_SetActiveVolumeUnit.vi"("error in (no error)"=w89, "active volume unit"=1, "dosingunit"=w107, "device handle in"=w88) -> ("error out"=w110:errorcluster, "device handle out"=w111:u32)
    n9 = call "NCS_SetActiveFlowUnit.vi"("error in (no error)"=w110, "active flow unit"=3, "dosingunit"=w107, "device handle in"=w111) -> ("error out"=w108:errorcluster, "device handle out"=w109:u32)
    n10 = call "NCS_GetSyringeLevelMax.vi"("error in (no error)"=w108, "dosingunit"=w107, "device handle in"=w109) -> ("error out"=w105:errorcluster, "syringe level max"=w104:dbl, "device handle out"=w106:u32)  [unwired: 1 out]
    n11 = call "NCS_GetFlowRateMax.vi"("error in (no error)"=w105, "dosingunit"=w107, "device handle in"=w106) -> ("error out"=w92:errorcluster, "device handle out"=w93:u32)  [unwired: 1 out]
    n12 = call "NCS_GetActiveFlowUnit.vi"("error in (no error)"=w92, "device handle in"=w93) -> ("error out"=w100:errorcluster, "active flow unit"=w99:u8, "device handle out"=w101:u32)  [unwired: 1 in]
    n13 = call "NCS_GetFlowUnitString.vi"("device handle in"=w101, "flow unit id"=w99, "error in (no error)"=w100) -> ("device handle out"=w96:u32, "error out"=w95:errorcluster)  [unwired: 2 out]
    n14 = call "NCS_GetActiveVolumeUnit.vi"("error in (no error)"=w95, "device handle in"=w96) -> ("error out"=w97:errorcluster, "active volume unit"=w98:u8, "device handle out"=w94:u32)  [unwired: 1 in]
    n15 = call "NCS_GetVolumeUnitString.vi"("device handle in"=w94, "volume unit id"=w98, "error in (no error)"=w97) -> ("device handle out"=w91:u32, "error out"=w90:errorcluster)  [unwired: 2 out]
  }
  n16 = call-poly <vilib>:"DAQmx Create Virtual Channel.vi"("maximum value"=10.0, "minimum value"=-10.0 ("maximum value"), "input terminal configuration"="Liquid P sensor Terminal Configuration", "physical channels"="Liquid P sensor Physical Channel") -> ("task out"=w44:refnum<k21>, "error out"=w45:errorcluster)  [unwired: 10 in]
  n17 = Current VI's Path() -> (path=w57:path)
  n18 = Strip Path(path=w57) -> (stripped path=w56:path)  [unwired: 1 out]
  n19 = call <vilib>:"DAQmx Start Task.vi"("task/channels in"=w44, "error in"=w45) -> ("task out"=w43:refnum<k21>, "error out"=w42:errorcluster)  [unwired: 12 in]
  n20 = Build Path(base path=w56, name or relative path="pcal.txt") -> (appended path=w15:path)
  n21 = Scan From String(w15, w16) -> (w14:errorcluster, output 1=w13:dbl, output 2=w12:dbl, output 3=w11:dbl, output 4=w10:dbl, output 5=w9:dbl, output 6=w8:dbl, output 7=w7:dbl, output 8=w6:dbl)  [unwired: 9 in, 1 out]
  "Slope 1" <- w13
  "Intercept 1" <- w12
  "Intercept 2" <- w10
  "Intercept  3" <- w8
  "Intercept 4" <- w6
  "Slope 2" <- w11
  "Slope 3" <- w9
  "Slope 4" <- w7
  n22 = call "CN7500_Initialize.vi"("VISA resource name"=refnum<visa-resource-name> "COM8") -> ("error out"=w72:errorcluster, "VISA resource name out"=w73:refnum<visa-resource-name>)  [unwired: 9 in]
  n23 = call "CN7500_Write Set Point Value.vi"("Target Set Point Value"=25.0, "error in (no error)"=w72, "Controller Number"=w66, "VISA In"=w73) -> ("error out"=w64:errorcluster, "VISA Out"=w65:refnum<visa-resource-name>)  [unwired: 6 in]
  n24 = call <vilib>:"DAQmx Start Task.vi"("task/channels in"=w48, "error in"=w14) -> ("task out"=w54:refnum<k21>, "error out"=w53:errorcluster)  [unwired: 12 in]
  n25 = Divide(x="Conc NaOH in Syringe", y=2) -> (x/y=w3:dbl)
  n26 = while {
    tunnel: w81 -> [w166]
    tunnel: w80 -> [w165]
    tunnel: [w164] -> w75
    tunnel: [w163] -> w74
    tunnel: w66 -> [w160]
    tunnel: w65 -> [w159]
    tunnel: w64 -> [w158]
    tunnel: [w157] -> w63
    tunnel: [w156] -> w62
    tunnel: w54 -> [w154]
    tunnel: w53 -> [w153]
    tunnel: w13 -> [w152]
    tunnel: w12 -> [w151]
    tunnel: [w150] -> w50
    tunnel: [w149] -> w49
    tunnel: w43 -> [w133]
    tunnel: w42 -> [w132]
    tunnel: [w131] -> w40
    tunnel: [w130] -> w38
    tunnel: w3 -> [w126]
    tunnel: "Cat Mass mg" -> [w125]
    tunnel: w11 -> [w124]
    tunnel: w10 -> [w123]
    tunnel: w9 -> [w122]
    tunnel: w8 -> [w121]
    tunnel: w7 -> [w120]
    tunnel: w6 -> [w119]
    tunnel: "Total Gas Flow Rate" -> [w118]
    tunnel: "Back Pressure Bar Abs" -> [w117]
    i -> [w143]
    stop <- w148 stop-if-true
    # "Should be in formats \nMBDoE\nC:\\\\Users\\\\User\\\\Documents\\\\LabVIEW Data\\\\2015 Projects\\\\Combined\\Recordfilelabfirst.xlsx"
    n27 = node-c288() -> (w162:T1)  [unwired: 4 in]
    n28 = case shown="False" "Automated Experiments or Direct Control" {
      tunnel: [w187 w866] -> w146
      tunnel: [w185 w866] -> w145
      tunnel: [w189 w866] -> w144
      tunnel: w143 -> [w190 _]
      tunnel: "Conc 0  (M)" -> [w188 _]
      tunnel: "Flow 0" -> [w184 _]
      tunnel: "Temp 0" -> [w186 _]
      tunnel: "Temp 1" -> [w182 _]
      tunnel: "Flow 1" -> [w181 _]
      tunnel: "Conc 1" -> [w180 _]
      tunnel: "HPLC file Name -doesnt need extension" -> [w179 _]
      tunnel: "Result file name -  needs extension RecordHMF.xlsx" -> [w183 _]
      tunnel: "Temp 2" -> [w178 _]
      tunnel: "Flow 2" -> [w177 _]
      tunnel: "Conc 2" -> [w176 _]
      tunnel: w126 -> [w175 _]
      tunnel: w125 -> [w174 _]
      tunnel: w118 -> [w173 w864]
      tunnel: w117 -> [w172 _]
      tunnel: "O2 frac 1" -> [w171 _]
      tunnel: "O2 frac 2" -> [w170 _]
      tunnel: "O2 frac 0" -> [w169 w865]
      tunnel: [w168 w865] -> w113
      tunnel: [w167 w864] -> w112
      frame False {
        # "o2 fraction"
        n29 = case shown="4" w190 {
          tunnel: [w194 w199 w220 w253 w336 w419 w502 w585 w668 w751 w830] -> w189
          tunnel: w188 -> [w194 _ _ _ _ _ _ _ _ _ w830]
          tunnel: [w196 w201 w229 w248 w338 w421 w504 w587 w670 w753 w832] -> w187
          tunnel: w186 -> [w196 _ _ _ _ _ _ _ _ _ w832]
          tunnel: [w195 w200 w228 w249 w337 w420 w503 w586 w669 w752 w831] -> w185
          tunnel: w184 -> [w195 _ _ _ _ _ _ _ _ _ w831]
          tunnel: w183 -> [_ _ w230 w254 w335 w418 w501 w584 w667 w750 w829]
          tunnel: w182 -> [_ w201 w229 _ _ _ _ _ _ _ _]
          tunnel: w181 -> [_ w200 w228 _ _ _ _ _ _ _ _]
          tunnel: w180 -> [_ w199 w220 _ _ _ _ _ _ _ _]
          tunnel: w179 -> [_ _ _ w255 w339 w422 w505 w588 w671 w754 w833]
          tunnel: w178 -> [_ _ _ w248 _ _ _ _ _ _ _]
          tunnel: w177 -> [_ _ _ w249 _ _ _ _ _ _ _]
          tunnel: w176 -> [_ _ _ w253 _ _ _ _ _ _ _]
          tunnel: w175 -> [_ _ w219 w252 w333 w416 w499 w582 w665 w748 _]
          tunnel: w174 -> [_ _ w205 w250 w332 w415 w498 w581 w664 w747 _]
          tunnel: w173 -> [w191 w197 w203 w246 w330 w412 w496 w578 w662 w744 w827]
          tunnel: w172 -> [_ _ w218 w251 w331 w414 w497 w580 w663 w746 _]
          tunnel: w171 -> [_ w198 w204 _ _ _ _ _ _ _ _]
          tunnel: w170 -> [_ _ _ w247 _ _ _ _ _ _ _]
          tunnel: [w192 w198 w204 w247 w329 w413 w495 w579 w661 w745 w828] -> w168
          tunnel: w169 -> [w192 _ _ _ _ _ _ _ _ _ w828]
          tunnel: [w191 w197 w203 w246 w330 w412 w496 w578 w662 w744 w827] -> w167
          frame 0, Default {
            (unwired) 0
            "Exp 0" <- TRUE
          }
          frame 1 {
            (unwired) 0
            # "total gas flowrate"
            "Exp 2" <- TRUE
          }
          frame 2 {
            # "cat mass"
            # "C H"
            # "C N"
            # "G"
            # "P"
            # "Y"
            # "L"
            # "T"
            n30 = call <vilib>:"New Session.vi"("Path to Python Module (.py File)"=path "C:/Users/User/Documents/LabVIEW Data/2015 Projects/Combined/WriteHMFInputs.py") -> ("error out"=w237:errorcluster, "Session ID out"=w236:T4)  [unwired: 9 in]
            n31 = call <vilib>:"Pack.vi"("Argument"=w230, "error in (no error)"=w237, "Session ID"=w236) -> ("error out"=w238:errorcluster, "Python Object References Out"=w242:T5, "Session ID out"=w235:T4)  [unwired: 6 in]
            n32 = call <vilib>:"Pack.vi"("Argument"=w229, "error in (no error)"=w238, "Python Object References In"=w242, "Session ID"=w235) -> ("error out"=w239:errorcluster, "Python Object References Out"=w243:T5, "Session ID out"=w245:T4)  [unwired: 5 in]
            n33 = call <vilib>:"Pack.vi"("Argument"=w228, "error in (no error)"=w239, "Python Object References In"=w243, "Session ID"=w245) -> ("error out"=w240:errorcluster, "Python Object References Out"=w244:T5, "Session ID out"=w231:T4)  [unwired: 5 in]
            n34 = call <vilib>:"Pack.vi"("Argument"=w203, "error in (no error)"=w240, "Python Object References In"=w244, "Session ID"=w231) -> ("error out"=w222:errorcluster, "Python Object References Out"=w224:T5, "Session ID out"=w226:T4)  [unwired: 5 in]
            n35 = call <vilib>:"Pack.vi"("Argument"=w220, "error in (no error)"=w222, "Python Object References In"=w224, "Session ID"=w226) -> ("error out"=w221:errorcluster, "Python Object References Out"=w223:T5, "Session ID out"=w225:T4)  [unwired: 5 in]
            n36 = call <vilib>:"Pack.vi"("Argument"=w219, "error in (no error)"=w221, "Python Object References In"=w223, "Session ID"=w225) -> ("error out"=w217:errorcluster, "Python Object References Out"=w213:T5, "Session ID out"=w209:T4)  [unwired: 5 in]
            n37 = call <vilib>:"Pack.vi"("Argument"=w218, "error in (no error)"=w217, "Python Object References In"=w213, "Session ID"=w209) -> ("error out"=w216:errorcluster, "Python Object References Out"=w212:T5, "Session ID out"=w208:T4)  [unwired: 5 in]
            n38 = call <vilib>:"Pack.vi"("Argument"=w204, "error in (no error)"=w216, "Python Object References In"=w212, "Session ID"=w208) -> ("error out"=w215:errorcluster, "Python Object References Out"=w211:T5, "Session ID out"=w207:T4)  [unwired: 5 in]
            n39 = call <vilib>:"Pack.vi"("Argument"=w205, "error in (no error)"=w215, "Python Object References In"=w211, "Session ID"=w207) -> ("error out"=w214:errorcluster, "Python Object References Out"=w210:T5, "Session ID out"=w206:T4)  [unwired: 5 in]
            n40 = call <vilib>:"Call.vi"("Function or Method Name"="AppendResultFile", "error in (no error)"=w214, "Python Object References In"=w210, "Session ID"=w206) -> ("error out"=w241:errorcluster, "Session ID out"=w232:T4)  [unwired: 5 in, 1 out]
            n41 = call <vilib>:"Close Session.vi"("error in (no error)"=w241, "Session ID"=w232) -> ()  [unwired: 9 in, 1 out]
            "Temp 1" <- w229
            "Flow 1" <- w228
            "Conc 1" <- w220
            "Exp 1" <- TRUE
            "O2 frac 1" <- w204
          }
          frame 3 {
            n42 = flat-sequence {
              tunnel: w255 -> [w258]
              tunnel: w254 -> [w257]
              tunnel: w254 -> [w295]
              tunnel: w248 -> [w287]
              tunnel: w249 -> [w294]
              tunnel: w246 -> [w293]
              tunnel: w253 -> [w292]
              tunnel: w252 -> [w291]
              tunnel: w251 -> [w290]
              tunnel: w250 -> [w289]
              tunnel: w247 -> [w288]
              frame #0 {
                n43 = call <vilib>:"New Session.vi"("Path to Python Module (.py File)"=path "C:/Users/User/Documents/LabVIEW Data/2015 Projects/Combined/HMF_onlineHPLC.py") -> ("error out"=w284:errorcluster, "Session ID out"=w283:T4)  [unwired: 9 in]
                n44 = call <vilib>:"Pack.vi"("Argument"=w258, "error in (no error)"=w284, "Session ID"=w283) -> ("error out"=w270:errorcluster, "Python Object References Out"=w272:T5, "Session ID out"=w274:T4)  [unwired: 6 in]
                n45 = call <vilib>:"Pack.vi"("Argument"=w257, "error in (no error)"=w270, "Python Object References In"=w272, "Session ID"=w274) -> ("error out"=w269:errorcluster, "Python Object References Out"=w271:T5, "Session ID out"=w273:T4)  [unwired: 5 in]
                n46 = call <vilib>:"Call.vi"("Function or Method Name"="HPLC", "error in (no error)"=w269, "Python Object References In"=w271, "Session ID"=w273) -> ("error out"=w285:errorcluster, "Python Object References Out"=w277:T5, "Session ID out"=w278:T4)  [unwired: 5 in]
                n47 = call-poly <vilib>:"Unpack.vi"("error in (no error)"=w285, "Python Object References In"=w277, "Session ID"=w278) -> ("error out"=w286:errorcluster, "Value"=→"C HMF 1":dbl, "Python Object References Out"=w282:T5, "Session ID out"=w281:T4)  [unwired: 5 in]
                n48 = call-poly <vilib>:"Unpack.vi"("error in (no error)"=w286, "Python Object References In"=w282, "Session ID"=w281) -> ("error out"=w261:errorcluster, "Value"=→"C HFCA 1":dbl, "Python Object References Out"=w262:T5, "Session ID out"=w263:T4)  [unwired: 5 in]
                n49 = call-poly <vilib>:"Unpack.vi"("error in (no error)"=w261, "Python Object References In"=w262, "Session ID"=w263) -> ("error out"=w268:errorcluster, "Value"=→"C FFCA 1":dbl, "Python Object References Out"=w267:T5, "Session ID out"=w266:T4)  [unwired: 5 in]
                n50 = call-poly <vilib>:"Unpack.vi"("error in (no error)"=w268, "Python Object References In"=w267, "Session ID"=w266) -> ("error out"=w259:errorcluster, "Value"=→"C FDCA 1":dbl, "Session ID out"=w260:T4)  [unwired: 5 in, 1 out]
                n51 = call <vilib>:"Close Session.vi"("error in (no error)"=w259, "Session ID"=w260) -> ()  [unwired: 9 in, 1 out]
              }
              frame #1 {
                # "cat mass"
                # "C H"
                # "C N"
                # "G"
                # "P"
                # "Y"
                # "L"
                # "T"
                n52 = call <vilib>:"New Session.vi"("Path to Python Module (.py File)"=path "C:/Users/User/Documents/LabVIEW Data/2015 Projects/Combined/WriteHMFInputs.py") -> ("error out"=w304:errorcluster, "Session ID out"=w305:T4)  [unwired: 9 in]
                n53 = call <vilib>:"Pack.vi"("Argument"=w295, "error in (no error)"=w304, "Session ID"=w305) -> ("error out"=w303:errorcluster, "Python Object References Out"=w299:T5, "Session ID out"=w306:T4)  [unwired: 6 in]
                n54 = call <vilib>:"Pack.vi"("Argument"=w287, "error in (no error)"=w303, "Python Object References In"=w299, "Session ID"=w306) -> ("error out"=w302:errorcluster, "Python Object References Out"=w298:T5, "Session ID out"=w296:T4)  [unwired: 5 in]
                n55 = call <vilib>:"Pack.vi"("Argument"=w294, "error in (no error)"=w302, "Python Object References In"=w298, "Session ID"=w296) -> ("error out"=w301:errorcluster, "Python Object References Out"=w297:T5, "Session ID out"=w310:T4)  [unwired: 5 in]
                n56 = call <vilib>:"Pack.vi"("Argument"=w293, "error in (no error)"=w301, "Python Object References In"=w297, "Session ID"=w310) -> ("error out"=w315:errorcluster, "Python Object References Out"=w313:T5, "Session ID out"=w311:T4)  [unwired: 5 in]
                n57 = call <vilib>:"Pack.vi"("Argument"=w292, "error in (no error)"=w315, "Python Object References In"=w313, "Session ID"=w311) -> ("error out"=w316:errorcluster, "Python Object References Out"=w314:T5, "Session ID out"=w312:T4)  [unwired: 5 in]
                n58 = call <vilib>:"Pack.vi"("Argument"=w291, "error in (no error)"=w316, "Python Object References In"=w314, "Session ID"=w312) -> ("error out"=w317:errorcluster, "Python Object References Out"=w321:T5, "Session ID out"=w325:T4)  [unwired: 5 in]
                n59 = call <vilib>:"Pack.vi"("Argument"=w290, "error in (no error)"=w317, "Python Object References In"=w321, "Session ID"=w325) -> ("error out"=w318:errorcluster, "Python Object References Out"=w322:T5, "Session ID out"=w326:T4)  [unwired: 5 in]
                n60 = call <vilib>:"Pack.vi"("Argument"=w288, "error in (no error)"=w318, "Python Object References In"=w322, "Session ID"=w326) -> ("error out"=w319:errorcluster, "Python Object References Out"=w323:T5, "Session ID out"=w327:T4)  [unwired: 5 in]
                n61 = call <vilib>:"Pack.vi"("Argument"=w289, "error in (no error)"=w319, "Python Object References In"=w323, "Session ID"=w327) -> ("error out"=w320:errorcluster, "Python Object References Out"=w324:T5, "Session ID out"=w328:T4)  [unwired: 5 in]
                n62 = call <vilib>:"Call.vi"("Function or Method Name"="AppendResultFile", "error in (no error)"=w320, "Python Object References In"=w324, "Session ID"=w328) -> ("error out"=w300:errorcluster, "Session ID out"=w309:T4)  [unwired: 5 in, 1 out]
                n63 = call <vilib>:"Close Session.vi"("error in (no error)"=w300, "Session ID"=w309) -> ()  [unwired: 9 in, 1 out]
                "Temp 2" <- w287
                "Flow 2" <- w294
                "Conc 2" <- w292
                "O2 frac 2" <- w288
              }
            }
            "Exp 9" <- TRUE
          }
          frame 4 {
            n64 = flat-sequence {
              tunnel: w339 -> [w357]
              tunnel: w335 -> [w350]
              tunnel: w335 -> [_]
              tunnel: w335 -> [w378]
              tunnel: ["Temp 3"] -> w338
              tunnel: ["Flow 3"] -> w337
              tunnel: ["Conc 3"] -> w336
              tunnel: w333 -> [w373]
              tunnel: w332 -> [w371]
              tunnel: w330 -> [w374]
              tunnel: w331 -> [w372]
              tunnel: ["O2 frac3"] -> w329
              frame #0 {
                # "make this include a write to record file step"
                n65 = call <vilib>:"New Session.vi"("Path to Python Module (.py File)"=path "C:/Users/User/Documents/LabVIEW Data/2015 Projects/Combined/HMF_onlineHPLC.py") -> ("error out"=w367:errorcluster, "Session ID out"=w366:T4)  [unwired: 9 in]
                n66 = call <vilib>:"Pack.vi"("Argument"=w357, "error in (no error)"=w367, "Session ID"=w366) -> ("error out"=w352:errorcluster, "Python Object References Out"=w354:T5, "Session ID out"=w356:T4)  [unwired: 6 in]
                n67 = call <vilib>:"Pack.vi"("Argument"=w350, "error in (no error)"=w352, "Python Object References In"=w354, "Session ID"=w356) -> ("error out"=w351:errorcluster, "Python Object References Out"=w353:T5, "Session ID out"=w355:T4)  [unwired: 5 in]
                n68 = call <vilib>:"Call.vi"("Function or Method Name"="HPLC", "error in (no error)"=w351, "Python Object References In"=w353, "Session ID"=w355) -> ("error out"=w368:errorcluster, "Python Object References Out"=w360:T5, "Session ID out"=w361:T4)  [unwired: 5 in]
                n69 = call-poly <vilib>:"Unpack.vi"("error in (no error)"=w368, "Python Object References In"=w360, "Session ID"=w361) -> ("error out"=w369:errorcluster, "Value"=→"C HMF 2":dbl, "Python Object References Out"=w365:T5, "Session ID out"=w364:T4)  [unwired: 5 in]
                n70 = call-poly <vilib>:"Unpack.vi"("error in (no error)"=w369, "Python Object References In"=w365, "Session ID"=w364) -> ("error out"=w341:errorcluster, "Value"=→"C HFCA 2":dbl, "Python Object References Out"=w340:T5, "Session ID out"=w342:T4)  [unwired: 5 in]
                n71 = call-poly <vilib>:"Unpack.vi"("error in (no error)"=w341, "Python Object References In"=w340, "Session ID"=w342) -> ("error out"=w349:errorcluster, "Value"=→"C FFCA 2":dbl, "Python Object References Out"=w348:T5, "Session ID out"=w347:T4)  [unwired: 5 in]
                n72 = call-poly <vilib>:"Unpack.vi"("error in (no error)"=w349, "Python Object References In"=w348, "Session ID"=w347) -> ("error out"=w343:errorcluster, "Value"=→"C FDCA 2":dbl, "Session ID out"=w344:T4)  [unwired: 5 in, 1 out]
                n73 = call <vilib>:"Close Session.vi"("error in (no error)"=w343, "Session ID"=w344) -> ()  [unwired: 9 in, 1 out]
              }
              frame #1 {
              }
              frame #2 {
                # "cat mass"
                # "C H"
                # "C N"
                # "G"
                # "P"
                # "Y"
                # "L"
                # "T"
                n74 = call <vilib>:"New Session.vi"("Path to Python Module (.py File)"=path "C:/Users/User/Documents/LabVIEW Data/2015 Projects/Combined/WriteHMFInputs.py") -> ("error out"=w403:errorcluster, "Session ID out"=w402:T4)  [unwired: 9 in]
                n75 = call <vilib>:"Pack.vi"("Argument"=w378, "error in (no error)"=w403, "Session ID"=w402) -> ("error out"=w404:errorcluster, "Python Object References Out"=w408:T5, "Session ID out"=w401:T4)  [unwired: 6 in]
                n76 = call <vilib>:"Pack.vi"("Argument"="Temp 3", "error in (no error)"=w404, "Python Object References In"=w408, "Session ID"=w401) -> ("error out"=w405:errorcluster, "Python Object References Out"=w409:T5, "Session ID out"=w411:T4)  [unwired: 5 in]
                n77 = call <vilib>:"Pack.vi"("Argument"="Flow 3", "error in (no error)"=w405, "Python Object References In"=w409, "Session ID"=w411) -> ("error out"=w406:errorcluster, "Python Object References Out"=w410:T5, "Session ID out"=w398:T4)  [unwired: 5 in]
                n78 = call <vilib>:"Pack.vi"("Argument"=w374, "error in (no error)"=w406, "Python Object References In"=w410, "Session ID"=w398) -> ("error out"=w393:errorcluster, "Python Object References Out"=w395:T5, "Session ID out"=w397:T4)  [unwired: 5 in]
                n79 = call <vilib>:"Pack.vi"("Argument"="Conc 3", "error in (no error)"=w393, "Python Object References In"=w395, "Session ID"=w397) -> ("error out"=w392:errorcluster, "Python Object References Out"=w394:T5, "Session ID out"=w396:T4)  [unwired: 5 in]
                n80 = call <vilib>:"Pack.vi"("Argument"=w373, "error in (no error)"=w392, "Python Object References In"=w394, "Session ID"=w396) -> ("error out"=w391:errorcluster, "Python Object References Out"=w387:T5, "Session ID out"=w383:T4)  [unwired: 5 in]
                n81 = call <vilib>:"Pack.vi"("Argument"=w372, "error in (no error)"=w391, "Python Object References In"=w387, "Session ID"=w383) -> ("error out"=w390:errorcluster, "Python Object References Out"=w386:T5, "Session ID out"=w382:T4)  [unwired: 5 in]
                n82 = call <vilib>:"Pack.vi"("Argument"="O2 frac3", "error in (no error)"=w390, "Python Object References In"=w386, "Session ID"=w382) -> ("error out"=w389:errorcluster, "Python Object References Out"=w385:T5, "Session ID out"=w381:T4)  [unwired: 5 in]
                n83 = call <vilib>:"Pack.vi"("Argument"=w371, "error in (no error)"=w389, "Python Object References In"=w385, "Session ID"=w381) -> ("error out"=w388:errorcluster, "Python Object References Out"=w384:T5, "Session ID out"=w380:T4)  [unwired: 5 in]
                n84 = call <vilib>:"Call.vi"("Function or Method Name"="AppendResultFile", "error in (no error)"=w388, "Python Object References In"=w384, "Session ID"=w380) -> ("error out"=w407:errorcluster, "Session ID out"=w399:T4)  [unwired: 5 in, 1 out]
                n85 = call <vilib>:"Close Session.vi"("error in (no error)"=w407, "Session ID"=w399) -> ()  [unwired: 9 in, 1 out]
                "Temp 3" <- "Temp 3"
                "Flow 3" <- "Flow 3"
                "Conc 3" <- "Conc 3"
                "O2 frac 3" <- "O2 frac3"
              }
            }
            "Exp 3" <- TRUE
          }
          frame 5 {
            n86 = flat-sequence {
              tunnel: w422 -> [w440]
              tunnel: w418 -> [w433]
              tunnel: w418 -> [_]
              tunnel: w418 -> [w461]
              tunnel: ["Temp 4"] -> w421
              tunnel: ["Flow 4"] -> w420
              tunnel: ["Conc 4"] -> w419
              tunnel: w416 -> [w456]
              tunnel: w415 -> [w454]
              tunnel: w412 -> [w458]
              tunnel: w414 -> [w455]
              tunnel: ["O2 frac 4"] -> w413
              frame #0 {
                # "make this include a write to record file step"
                n87 = call <vilib>:"New Session.vi"("Path to Python Module (.py File)"=path "C:/Users/User/Documents/LabVIEW Data/2015 Projects/Combined/HMF_onlineHPLC.py") -> ("error out"=w450:errorcluster, "Session ID out"=w449:T4)  [unwired: 9 in]
                n88 = call <vilib>:"Pack.vi"("Argument"=w440, "error in (no error)"=w450, "Session ID"=w449) -> ("error out"=w435:errorcluster, "Python Object References Out"=w437:T5, "Session ID out"=w439:T4)  [unwired: 6 in]
                n89 = call <vilib>:"Pack.vi"("Argument"=w433, "error in (no error)"=w435, "Python Object References In"=w437, "Session ID"=w439) -> ("error out"=w434:errorcluster, "Python Object References Out"=w436:T5, "Session ID out"=w438:T4)  [unwired: 5 in]
                n90 = call <vilib>:"Call.vi"("Function or Method Name"="HPLC", "error in (no error)"=w434, "Python Object References In"=w436, "Session ID"=w438) -> ("error out"=w451:errorcluster, "Python Object References Out"=w443:T5, "Session ID out"=w444:T4)  [unwired: 5 in]
                n91 = call-poly <vilib>:"Unpack.vi"("error in (no error)"=w451, "Python Object References In"=w443, "Session ID"=w444) -> ("error out"=w452:errorcluster, "Value"=→"C HMF 3":dbl, "Python Object References Out"=w448:T5, "Session ID out"=w447:T4)  [unwired: 5 in]
                n92 = call-poly <vilib>:"Unpack.vi"("error in (no error)"=w452, "Python Object References In"=w448, "Session ID"=w447) -> ("error out"=w424:errorcluster, "Value"=→"C HFCA 3":dbl, "Python Object References Out"=w423:T5, "Session ID out"=w425:T4)  [unwired: 5 in]
                n93 = call-poly <vilib>:"Unpack.vi"("error in (no error)"=w424, "Python Object References In"=w423, "Session ID"=w425) -> ("error out"=w432:errorcluster, "Value"=→"C FFCA 3":dbl, "Python Object References Out"=w431:T5, "Session ID out"=w430:T4)  [unwired: 5 in]
                n94 = call-poly <vilib>:"Unpack.vi"("error in (no error)"=w432, "Python Object References In"=w431, "Session ID"=w430) -> ("error out"=w426:errorcluster, "Value"=→"C FDCA 3":dbl, "Session ID out"=w427:T4)  [unwired: 5 in, 1 out]
                n95 = call <vilib>:"Close Session.vi"("error in (no error)"=w426, "Session ID"=w427) -> ()  [unwired: 9 in, 1 out]
              }
              frame #1 {
              }
              frame #2 {
                # "cat mass"
                # "C H"
                # "C N"
                # "G"
                # "P"
                # "Y"
                # "L"
                # "T"
                n96 = call <vilib>:"New Session.vi"("Path to Python Module (.py File)"=path "C:/Users/User/Documents/LabVIEW Data/2015 Projects/Combined/WriteHMFInputs.py") -> ("error out"=w486:errorcluster, "Session ID out"=w485:T4)  [unwired: 9 in]
                n97 = call <vilib>:"Pack.vi"("Argument"=w461, "error in (no error)"=w486, "Session ID"=w485) -> ("error out"=w487:errorcluster, "Python Object References Out"=w491:T5, "Session ID out"=w484:T4)  [unwired: 6 in]
                n98 = call <vilib>:"Pack.vi"("Argument"="Temp 4", "error in (no error)"=w487, "Python Object References In"=w491, "Session ID"=w484) -> ("error out"=w488:errorcluster, "Python Object References Out"=w492:T5, "Session ID out"=w494:T4)  [unwired: 5 in]
                n99 = call <vilib>:"Pack.vi"("Argument"="Flow 4", "error in (no error)"=w488, "Python Object References In"=w492, "Session ID"=w494) -> ("error out"=w489:errorcluster, "Python Object References Out"=w493:T5, "Session ID out"=w481:T4)  [unwired: 5 in]
                n100 = call <vilib>:"Pack.vi"("Argument"=w458, "error in (no error)"=w489, "Python Object References In"=w493, "Session ID"=w481) -> ("error out"=w476:errorcluster, "Python Object References Out"=w478:T5, "Session ID out"=w480:T4)  [unwired: 5 in]
                n101 = call <vilib>:"Pack.vi"("Argument"="Conc 4", "error in (no error)"=w476, "Python Object References In"=w478, "Session ID"=w480) -> ("error out"=w475:errorcluster, "Python Object References Out"=w477:T5, "Session ID out"=w479:T4)  [unwired: 5 in]
                n102 = call <vilib>:"Pack.vi"("Argument"=w456, "error in (no error)"=w475, "Python Object References In"=w477, "Session ID"=w479) -> ("error out"=w474:errorcluster, "Python Object References Out"=w470:T5, "Session ID out"=w466:T4)  [unwired: 5 in]
                n103 = call <vilib>:"Pack.vi"("Argument"=w455, "error in (no error)"=w474, "Python Object References In"=w470, "Session ID"=w466) -> ("error out"=w473:errorcluster, "Python Object References Out"=w469:T5, "Session ID out"=w465:T4)  [unwired: 5 in]
                n104 = call <vilib>:"Pack.vi"("Argument"="O2 frac 4", "error in (no error)"=w473, "Python Object References In"=w469, "Session ID"=w465) -> ("error out"=w472:errorcluster, "Python Object References Out"=w468:T5, "Session ID out"=w464:T4)  [unwired: 5 in]
                n105 = call <vilib>:"Pack.vi"("Argument"=w454, "error in (no error)"=w472, "Python Object References In"=w468, "Session ID"=w464) -> ("error out"=w471:errorcluster, "Python Object References Out"=w467:T5, "Session ID out"=w463:T4)  [unwired: 5 in]
                n106 = call <vilib>:"Call.vi"("Function or Method Name"="AppendResultFile", "error in (no error)"=w471, "Python Object References In"=w467, "Session ID"=w463) -> ("error out"=w490:errorcluster, "Session ID out"=w482:T4)  [unwired: 5 in, 1 out]
                n107 = call <vilib>:"Close Session.vi"("error in (no error)"=w490, "Session ID"=w482) -> ()  [unwired: 9 in, 1 out]
                "Temp 4" <- "Temp 4"
                "Flow 4" <- "Flow 4"
                "Conc 4" <- "Conc 4"
                "O2 frac 4" <- "O2 frac 4"
              }
            }
            "Exp 4" <- TRUE
          }
          frame 6 {
            n108 = flat-sequence {
              tunnel: w505 -> [w523]
              tunnel: w501 -> [w516]
              tunnel: w501 -> [_]
              tunnel: w501 -> [w544]
              tunnel: ["Temp 5"] -> w504
              tunnel: ["Flow 5"] -> w503
              tunnel: ["Conc 5"] -> w502
              tunnel: w499 -> [w539]
              tunnel: w498 -> [w537]
              tunnel: w496 -> [w541]
              tunnel: w497 -> [w538]
              tunnel: ["O2 frac 5"] -> w495
              frame #0 {
                # "make this include a write to record file step"
                n109 = call <vilib>:"New Session.vi"("Path to Python Module (.py File)"=path "C:/Users/User/Documents/LabVIEW Data/2015 Projects/Combined/HMF_onlineHPLC.py") -> ("error out"=w533:errorcluster, "Session ID out"=w532:T4)  [unwired: 9 in]
                n110 = call <vilib>:"Pack.vi"("Argument"=w523, "error in (no error)"=w533, "Session ID"=w532) -> ("error out"=w520:errorcluster, "Python Object References Out"=w521:T5, "Session ID out"=w522:T4)  [unwired: 6 in]
                n111 = call <vilib>:"Pack.vi"("Argument"=w516, "error in (no error)"=w520, "Python Object References In"=w521, "Session ID"=w522) -> ("error out"=w519:errorcluster, "Python Object References Out"=w518:T5, "Session ID out"=w517:T4)  [unwired: 5 in]
                n112 = call <vilib>:"Call.vi"("Function or Method Name"="HPLC", "error in (no error)"=w519, "Python Object References In"=w518, "Session ID"=w517) -> ("error out"=w534:errorcluster, "Python Object References Out"=w526:T5, "Session ID out"=w527:T4)  [unwired: 5 in]
                n113 = call-poly <vilib>:"Unpack.vi"("error in (no error)"=w534, "Python Object References In"=w526, "Session ID"=w527) -> ("error out"=w535:errorcluster, "Value"=→"C HMF 4":dbl, "Python Object References Out"=w531:T5, "Session ID out"=w530:T4)  [unwired: 5 in]
                n114 = call-poly <vilib>:"Unpack.vi"("error in (no error)"=w535, "Python Object References In"=w531, "Session ID"=w530) -> ("error out"=w507:errorcluster, "Value"=→"C HFCA 4":dbl, "Python Object References Out"=w506:T5, "Session ID out"=w508:T4)  [unwired: 5 in]
                n115 = call-poly <vilib>:"Unpack.vi"("error in (no error)"=w507, "Python Object References In"=w506, "Session ID"=w508) -> ("error out"=w515:errorcluster, "Value"=→"C FFCA 4":dbl, "Python Object References Out"=w514:T5, "Session ID out"=w513:T4)  [unwired: 5 in]
                n116 = call-poly <vilib>:"Unpack.vi"("error in (no error)"=w515, "Python Object References In"=w514, "Session ID"=w513) -> ("error out"=w509:errorcluster, "Value"=→"C FDCA 4":dbl, "Session ID out"=w510:T4)  [unwired: 5 in, 1 out]
                n117 = call <vilib>:"Close Session.vi"("error in (no error)"=w509, "Session ID"=w510) -> ()  [unwired: 9 in, 1 out]
              }
              frame #1 {
              }
              frame #2 {
                # "cat mass"
                # "C H"
                # "C N"
                # "G"
                # "P"
                # "Y"
                # "L"
                # "T"
                n118 = call <vilib>:"New Session.vi"("Path to Python Module (.py File)"=path "C:/Users/User/Documents/LabVIEW Data/2015 Projects/Combined/WriteHMFInputs.py") -> ("error out"=w569:errorcluster, "Session ID out"=w568:T4)  [unwired: 9 in]
                n119 = call <vilib>:"Pack.vi"("Argument"=w544, "error in (no error)"=w569, "Session ID"=w568) -> ("error out"=w570:errorcluster, "Python Object References Out"=w574:T5, "Session ID out"=w567:T4)  [unwired: 6 in]
                n120 = call <vilib>:"Pack.vi"("Argument"="Temp 5", "error in (no error)"=w570, "Python Object References In"=w574, "Session ID"=w567) -> ("error out"=w571:errorcluster, "Python Object References Out"=w575:T5, "Session ID out"=w577:T4)  [unwired: 5 in]
                n121 = call <vilib>:"Pack.vi"("Argument"="Flow 5", "error in (no error)"=w571, "Python Object References In"=w575, "Session ID"=w577) -> ("error out"=w572:errorcluster, "Python Object References Out"=w576:T5, "Session ID out"=w564:T4)  [unwired: 5 in]
                n122 = call <vilib>:"Pack.vi"("Argument"=w541, "error in (no error)"=w572, "Python Object References In"=w576, "Session ID"=w564) -> ("error out"=w559:errorcluster, "Python Object References Out"=w561:T5, "Session ID out"=w563:T4)  [unwired: 5 in]
                n123 = call <vilib>:"Pack.vi"("Argument"="Conc 5", "error in (no error)"=w559, "Python Object References In"=w561, "Session ID"=w563) -> ("error out"=w558:errorcluster, "Python Object References Out"=w560:T5, "Session ID out"=w562:T4)  [unwired: 5 in]
                n124 = call <vilib>:"Pack.vi"("Argument"=w539, "error in (no error)"=w558, "Python Object References In"=w560, "Session ID"=w562) -> ("error out"=w557:errorcluster, "Python Object References Out"=w553:T5, "Session ID out"=w549:T4)  [unwired: 5 in]
                n125 = call <vilib>:"Pack.vi"("Argument"=w538, "error in (no error)"=w557, "Python Object References In"=w553, "Session ID"=w549) -> ("error out"=w556:errorcluster, "Python Object References Out"=w552:T5, "Session ID out"=w548:T4)  [unwired: 5 in]
                n126 = call <vilib>:"Pack.vi"("Argument"="O2 frac 5", "error in (no error)"=w556, "Python Object References In"=w552, "Session ID"=w548) -> ("error out"=w555:errorcluster, "Python Object References Out"=w551:T5, "Session ID out"=w547:T4)  [unwired: 5 in]
                n127 = call <vilib>:"Pack.vi"("Argument"=w537, "error in (no error)"=w555, "Python Object References In"=w551, "Session ID"=w547) -> ("error out"=w554:errorcluster, "Python Object References Out"=w550:T5, "Session ID out"=w546:T4)  [unwired: 5 in]
                n128 = call <vilib>:"Call.vi"("Function or Method Name"="AppendResultFile", "error in (no error)"=w554, "Python Object References In"=w550, "Session ID"=w546) -> ("error out"=w573:errorcluster, "Session ID out"=w565:T4)  [unwired: 5 in, 1 out]
                n129 = call <vilib>:"Close Session.vi"("error in (no error)"=w573, "Session ID"=w565) -> ()  [unwired: 9 in, 1 out]
                "Temp 5" <- "Temp 5"
                "Flow 5" <- "Flow 5"
                "Conc 5" <- "Conc 5"
                "O2 frac 5" <- "O2 frac 5"
              }
            }
            "Exp 5" <- TRUE
          }
          frame 7 {
            n130 = flat-sequence {
              tunnel: w588 -> [w606]
              tunnel: w584 -> [w599]
              tunnel: w584 -> [_]
              tunnel: w584 -> [w627]
              tunnel: ["Temp 6"] -> w587
              tunnel: ["Flow 6"] -> w586
              tunnel: ["Conc 6"] -> w585
              tunnel: w582 -> [w622]
              tunnel: w581 -> [w620]
              tunnel: w578 -> [w624]
              tunnel: w580 -> [w621]
              tunnel: ["O2 frac 6"] -> w579
              frame #0 {
                # "make this include a write to record file step"
                n131 = call <vilib>:"New Session.vi"("Path to Python Module (.py File)"=path "C:/Users/User/Documents/LabVIEW Data/2015 Projects/Combined/HMF_onlineHPLC.py") -> ("error out"=w616:errorcluster, "Session ID out"=w615:T4)  [unwired: 9 in]
                n132 = call <vilib>:"Pack.vi"("Argument"=w606, "error in (no error)"=w616, "Session ID"=w615) -> ("error out"=w603:errorcluster, "Python Object References Out"=w604:T5, "Session ID out"=w605:T4)  [unwired: 6 in]
                n133 = call <vilib>:"Pack.vi"("Argument"=w599, "error in (no error)"=w603, "Python Object References In"=w604, "Session ID"=w605) -> ("error out"=w600:errorcluster, "Python Object References Out"=w601:T5, "Session ID out"=w602:T4)  [unwired: 5 in]
                n134 = call <vilib>:"Call.vi"("Function or Method Name"="HPLC", "error in (no error)"=w600, "Python Object References In"=w601, "Session ID"=w602) -> ("error out"=w617:errorcluster, "Python Object References Out"=w609:T5, "Session ID out"=w610:T4)  [unwired: 5 in]
                n135 = call-poly <vilib>:"Unpack.vi"("error in (no error)"=w617, "Python Object References In"=w609, "Session ID"=w610) -> ("error out"=w618:errorcluster, "Value"=→"C HMF 5":dbl, "Python Object References Out"=w614:T5, "Session ID out"=w613:T4)  [unwired: 5 in]
                n136 = call-poly <vilib>:"Unpack.vi"("error in (no error)"=w618, "Python Object References In"=w614, "Session ID"=w613) -> ("error out"=w590:errorcluster, "Value"=→"C HFCA 5":dbl, "Python Object References Out"=w589:T5, "Session ID out"=w591:T4)  [unwired: 5 in]
                n137 = call-poly <vilib>:"Unpack.vi"("error in (no error)"=w590, "Python Object References In"=w589, "Session ID"=w591) -> ("error out"=w598:errorcluster, "Value"=→"C FFCA 5":dbl, "Python Object References Out"=w597:T5, "Session ID out"=w596:T4)  [unwired: 5 in]
                n138 = call-poly <vilib>:"Unpack.vi"("error in (no error)"=w598, "Python Object References In"=w597, "Session ID"=w596) -> ("error out"=w592:errorcluster, "Value"=→"C FDCA 5":dbl, "Session ID out"=w593:T4)  [unwired: 5 in, 1 out]
                n139 = call <vilib>:"Close Session.vi"("error in (no error)"=w592, "Session ID"=w593) -> ()  [unwired: 9 in, 1 out]
              }
              frame #1 {
              }
              frame #2 {
                # "cat mass"
                # "C H"
                # "C N"
                # "G"
                # "P"
                # "Y"
                # "L"
                # "T"
                n140 = call <vilib>:"New Session.vi"("Path to Python Module (.py File)"=path "C:/Users/User/Documents/LabVIEW Data/2015 Projects/Combined/WriteHMFInputs.py") -> ("error out"=w652:errorcluster, "Session ID out"=w651:T4)  [unwired: 9 in]
                n141 = call <vilib>:"Pack.vi"("Argument"=w627, "error in (no error)"=w652, "Session ID"=w651) -> ("error out"=w653:errorcluster, "Python Object References Out"=w657:T5, "Session ID out"=w650:T4)  [unwired: 6 in]
                n142 = call <vilib>:"Pack.vi"("Argument"="Temp 6", "error in (no error)"=w653, "Python Object References In"=w657, "Session ID"=w650) -> ("error out"=w654:errorcluster, "Python Object References Out"=w658:T5, "Session ID out"=w660:T4)  [unwired: 5 in]
                n143 = call <vilib>:"Pack.vi"("Argument"="Flow 6", "error in (no error)"=w654, "Python Object References In"=w658, "Session ID"=w660) -> ("error out"=w655:errorcluster, "Python Object References Out"=w659:T5, "Session ID out"=w647:T4)  [unwired: 5 in]
                n144 = call <vilib>:"Pack.vi"("Argument"=w624, "error in (no error)"=w655, "Python Object References In"=w659, "Session ID"=w647) -> ("error out"=w642:errorcluster, "Python Object References Out"=w644:T5, "Session ID out"=w646:T4)  [unwired: 5 in]
                n145 = call <vilib>:"Pack.vi"("Argument"="Conc 6", "error in (no error)"=w642, "Python Object References In"=w644, "Session ID"=w646) -> ("error out"=w641:errorcluster, "Python Object References Out"=w643:T5, "Session ID out"=w645:T4)  [unwired: 5 in]
                n146 = call <vilib>:"Pack.vi"("Argument"=w622, "error in (no error)"=w641, "Python Object References In"=w643, "Session ID"=w645) -> ("error out"=w640:errorcluster, "Python Object References Out"=w636:T5, "Session ID out"=w632:T4)  [unwired: 5 in]
                n147 = call <vilib>:"Pack.vi"("Argument"=w621, "error in (no error)"=w640, "Python Object References In"=w636, "Session ID"=w632) -> ("error out"=w639:errorcluster, "Python Object References Out"=w635:T5, "Session ID out"=w631:T4)  [unwired: 5 in]
                n148 = call <vilib>:"Pack.vi"("Argument"="O2 frac 6", "error in (no error)"=w639, "Python Object References In"=w635, "Session ID"=w631) -> ("error out"=w638:errorcluster, "Python Object References Out"=w634:T5, "Session ID out"=w630:T4)  [unwired: 5 in]
                n149 = call <vilib>:"Pack.vi"("Argument"=w620, "error in (no error)"=w638, "Python Object References In"=w634, "Session ID"=w630) -> ("error out"=w637:errorcluster, "Python Object References Out"=w633:T5, "Session ID out"=w629:T4)  [unwired: 5 in]
                n150 = call <vilib>:"Call.vi"("Function or Method Name"="AppendResultFile", "error in (no error)"=w637, "Python Object References In"=w633, "Session ID"=w629) -> ("error out"=w656:errorcluster, "Session ID out"=w648:T4)  [unwired: 5 in, 1 out]
                n151 = call <vilib>:"Close Session.vi"("error in (no error)"=w656, "Session ID"=w648) -> ()  [unwired: 9 in, 1 out]
                "Temp 6" <- "Temp 6"
                "Flow 6" <- "Flow 6"
                "Conc 6" <- "Conc 6"
                "O2 frac 6" <- "O2 frac 6"
              }
            }
            "Exp 6" <- TRUE
          }
          frame 8 {
            n152 = flat-sequence {
              tunnel: w671 -> [w689]
              tunnel: w667 -> [w682]
              tunnel: w667 -> [_]
              tunnel: w667 -> [w710]
              tunnel: ["Temp 7"] -> w670
              tunnel: ["Flow 7"] -> w669
              tunnel: ["Conc 7"] -> w668
              tunnel: w665 -> [w705]
              tunnel: w664 -> [w703]
              tunnel: w662 -> [w707]
              tunnel: w663 -> [w704]
              tunnel: ["O2 frac 7"] -> w661
              frame #0 {
                n153 = call <vilib>:"New Session.vi"("Path to Python Module (.py File)"=path "C:/Users/User/Documents/LabVIEW Data/2015 Projects/Combined/HMF_onlineHPLC.py") -> ("error out"=w699:errorcluster, "Session ID out"=w698:T4)  [unwired: 9 in]
                n154 = call <vilib>:"Pack.vi"("Argument"=w689, "error in (no error)"=w699, "Session ID"=w698) -> ("error out"=w684:errorcluster, "Python Object References Out"=w686:T5, "Session ID out"=w688:T4)  [unwired: 6 in]
                n155 = call <vilib>:"Pack.vi"("Argument"=w682, "error in (no error)"=w684, "Python Object References In"=w686, "Session ID"=w688) -> ("error out"=w683:errorcluster, "Python Object References Out"=w685:T5, "Session ID out"=w687:T4)  [unwired: 5 in]
                n156 = call <vilib>:"Call.vi"("Function or Method Name"="HPLC", "error in (no error)"=w683, "Python Object References In"=w685, "Session ID"=w687) -> ("error out"=w700:errorcluster, "Python Object References Out"=w692:T5, "Session ID out"=w693:T4)  [unwired: 5 in]
                n157 = call-poly <vilib>:"Unpack.vi"("error in (no error)"=w700, "Python Object References In"=w692, "Session ID"=w693) -> ("error out"=w701:errorcluster, "Value"=→"C HMF 6":dbl, "Python Object References Out"=w697:T5, "Session ID out"=w696:T4)  [unwired: 5 in]
                n158 = call-poly <vilib>:"Unpack.vi"("error in (no error)"=w701, "Python Object References In"=w697, "Session ID"=w696) -> ("error out"=w673:errorcluster, "Value"=→"C HFCA 6":dbl, "Python Object References Out"=w672:T5, "Session ID out"=w674:T4)  [unwired: 5 in]
                n159 = call-poly <vilib>:"Unpack.vi"("error in (no error)"=w673, "Python Object References In"=w672, "Session ID"=w674) -> ("error out"=w681:errorcluster, "Value"=→"C FFCA 6":dbl, "Python Object References Out"=w680:T5, "Session ID out"=w679:T4)  [unwired: 5 in]
                n160 = call-poly <vilib>:"Unpack.vi"("error in (no error)"=w681, "Python Object References In"=w680, "Session ID"=w679) -> ("error out"=w675:errorcluster, "Value"=→"C FDCA 6":dbl, "Session ID out"=w676:T4)  [unwired: 5 in, 1 out]
                n161 = call <vilib>:"Close Session.vi"("error in (no error)"=w675, "Session ID"=w676) -> ()  [unwired: 9 in, 1 out]
              }
              frame #1 {
              }
              frame #2 {
                # "cat mass"
                # "C H"
                # "C N"
                # "G"
                # "P"
                # "Y"
                # "L"
                # "T"
                n162 = call <vilib>:"New Session.vi"("Path to Python Module (.py File)"=path "C:/Users/User/Documents/LabVIEW Data/2015 Projects/Combined/WriteHMFInputs.py") -> ("error out"=w735:errorcluster, "Session ID out"=w734:T4)  [unwired: 9 in]
                n163 = call <vilib>:"Pack.vi"("Argument"=w710, "error in (no error)"=w735, "Session ID"=w734) -> ("error out"=w736:errorcluster, "Python Object References Out"=w740:T5, "Session ID out"=w733:T4)  [unwired: 6 in]
                n164 = call <vilib>:"Pack.vi"("Argument"="Temp 7", "error in (no error)"=w736, "Python Object References In"=w740, "Session ID"=w733) -> ("error out"=w737:errorcluster, "Python Object References Out"=w741:T5, "Session ID out"=w743:T4)  [unwired: 5 in]
                n165 = call <vilib>:"Pack.vi"("Argument"="Flow 7", "error in (no error)"=w737, "Python Object References In"=w741, "Session ID"=w743) -> ("error out"=w738:errorcluster, "Python Object References Out"=w742:T5, "Session ID out"=w730:T4)  [unwired: 5 in]
                n166 = call <vilib>:"Pack.vi"("Argument"=w707, "error in (no error)"=w738, "Python Object References In"=w742, "Session ID"=w730) -> ("error out"=w725:errorcluster, "Python Object References Out"=w727:T5, "Session ID out"=w729:T4)  [unwired: 5 in]
                n167 = call <vilib>:"Pack.vi"("Argument"="Conc 7", "error in (no error)"=w725, "Python Object References In"=w727, "Session ID"=w729) -> ("error out"=w724:errorcluster, "Python Object References Out"=w726:T5, "Session ID out"=w728:T4)  [unwired: 5 in]
                n168 = call <vilib>:"Pack.vi"("Argument"=w705, "error in (no error)"=w724, "Python Object References In"=w726, "Session ID"=w728) -> ("error out"=w723:errorcluster, "Python Object References Out"=w719:T5, "Session ID out"=w715:T4)  [unwired: 5 in]
                n169 = call <vilib>:"Pack.vi"("Argument"=w704, "error in (no error)"=w723, "Python Object References In"=w719, "Session ID"=w715) -> ("error out"=w722:errorcluster, "Python Object References Out"=w718:T5, "Session ID out"=w714:T4)  [unwired: 5 in]
                n170 = call <vilib>:"Pack.vi"("Argument"="O2 frac 7", "error in (no error)"=w722, "Python Object References In"=w718, "Session ID"=w714) -> ("error out"=w721:errorcluster, "Python Object References Out"=w717:T5, "Session ID out"=w713:T4)  [unwired: 5 in]
                n171 = call <vilib>:"Pack.vi"("Argument"=w703, "error in (no error)"=w721, "Python Object References In"=w717, "Session ID"=w713) -> ("error out"=w720:errorcluster, "Python Object References Out"=w716:T5, "Session ID out"=w712:T4)  [unwired: 5 in]
                n172 = call <vilib>:"Call.vi"("Function or Method Name"="AppendResultFile", "error in (no error)"=w720, "Python Object References In"=w716, "Session ID"=w712) -> ("error out"=w739:errorcluster, "Session ID out"=w731:T4)  [unwired: 5 in, 1 out]
                n173 = call <vilib>:"Close Session.vi"("error in (no error)"=w739, "Session ID"=w731) -> ()  [unwired: 9 in, 1 out]
                "Temp 7" <- "Temp 7"
                "Flow 7" <- "Flow 7"
                "Conc 7" <- "Conc 7"
                "O2 frac 7" <- "O2 frac 7"
              }
            }
            "Exp 7" <- TRUE
          }
          frame 9 {
            n174 = flat-sequence {
              tunnel: w754 -> [w772]
              tunnel: w750 -> [w765]
              tunnel: w750 -> [_]
              tunnel: w750 -> [w793]
              tunnel: ["Temp 8"] -> w753
              tunnel: ["Flow 8"] -> w752
              tunnel: ["Conc 8"] -> w751
              tunnel: w748 -> [w788]
              tunnel: w747 -> [w786]
              tunnel: w744 -> [w790]
              tunnel: w746 -> [w787]
              tunnel: ["O2 frac 8"] -> w745
              frame #0 {
                n175 = call <vilib>:"New Session.vi"("Path to Python Module (.py File)"=path "C:/Users/User/Documents/LabVIEW Data/2015 Projects/Combined/HMF_onlineHPLC.py") -> ("error out"=w782:errorcluster, "Session ID out"=w781:T4)  [unwired: 9 in]
                n176 = call <vilib>:"Pack.vi"("Argument"=w772, "error in (no error)"=w782, "Session ID"=w781) -> ("error out"=w769:errorcluster, "Python Object References Out"=w770:T5, "Session ID out"=w771:T4)  [unwired: 6 in]
                n177 = call <vilib>:"Pack.vi"("Argument"=w765, "error in (no error)"=w769, "Python Object References In"=w770, "Session ID"=w771) -> ("error out"=w768:errorcluster, "Python Object References Out"=w767:T5, "Session ID out"=w766:T4)  [unwired: 5 in]
                n178 = call <vilib>:"Call.vi"("Function or Method Name"="HPLC", "error in (no error)"=w768, "Python Object References In"=w767, "Session ID"=w766) -> ("error out"=w783:errorcluster, "Python Object References Out"=w775:T5, "Session ID out"=w776:T4)  [unwired: 5 in]
                n179 = call-poly <vilib>:"Unpack.vi"("error in (no error)"=w783, "Python Object References In"=w775, "Session ID"=w776) -> ("error out"=w784:errorcluster, "Value"=→"C HMF 7":dbl, "Python Object References Out"=w780:T5, "Session ID out"=w779:T4)  [unwired: 5 in]
                n180 = call-poly <vilib>:"Unpack.vi"("error in (no error)"=w784, "Python Object References In"=w780, "Session ID"=w779) -> ("error out"=w756:errorcluster, "Value"=→"C HFCA 7":dbl, "Python Object References Out"=w755:T5, "Session ID out"=w757:T4)  [unwired: 5 in]
                n181 = call-poly <vilib>:"Unpack.vi"("error in (no error)"=w756, "Python Object References In"=w755, "Session ID"=w757) -> ("error out"=w764:errorcluster, "Value"=→"C FFCA 7":dbl, "Python Object References Out"=w763:T5, "Session ID out"=w762:T4)  [unwired: 5 in]
                n182 = call-poly <vilib>:"Unpack.vi"("error in (no error)"=w764, "Python Object References In"=w763, "Session ID"=w762) -> ("error out"=w758:errorcluster, "Value"=→"C FDCA 7":dbl, "Session ID out"=w759:T4)  [unwired: 5 in, 1 out]
                n183 = call <vilib>:"Close Session.vi"("error in (no error)"=w758, "Session ID"=w759) -> ()  [unwired: 9 in, 1 out]
              }
              frame #1 {
              }
              frame #2 {
                # "cat mass"
                # "C H"
                # "C N"
                # "G"
                # "P"
                # "Y"
                # "L"
                # "T"
                n184 = call <vilib>:"New Session.vi"("Path to Python Module (.py File)"=path "C:/Users/User/Documents/LabVIEW Data/2015 Projects/Combined/WriteHMFInputs.py") -> ("error out"=w818:errorcluster, "Session ID out"=w817:T4)  [unwired: 9 in]
                n185 = call <vilib>:"Pack.vi"("Argument"=w793, "error in (no error)"=w818, "Session ID"=w817) -> ("error out"=w819:errorcluster, "Python Object References Out"=w823:T5, "Session ID out"=w816:T4)  [unwired: 6 in]
                n186 = call <vilib>:"Pack.vi"("Argument"="Temp 8", "error in (no error)"=w819, "Python Object References In"=w823, "Session ID"=w816) -> ("error out"=w820:errorcluster, "Python Object References Out"=w824:T5, "Session ID out"=w826:T4)  [unwired: 5 in]
                n187 = call <vilib>:"Pack.vi"("Argument"="Flow 8", "error in (no error)"=w820, "Python Object References In"=w824, "Session ID"=w826) -> ("error out"=w821:errorcluster, "Python Object References Out"=w825:T5, "Session ID out"=w813:T4)  [unwired: 5 in]
                n188 = call <vilib>:"Pack.vi"("Argument"=w790, "error in (no error)"=w821, "Python Object References In"=w825, "Session ID"=w813) -> ("error out"=w808:errorcluster, "Python Object References Out"=w810:T5, "Session ID out"=w812:T4)  [unwired: 5 in]
                n189 = call <vilib>:"Pack.vi"("Argument"="Conc 8", "error in (no error)"=w808, "Python Object References In"=w810, "Session ID"=w812) -> ("error out"=w807:errorcluster, "Python Object References Out"=w809:T5, "Session ID out"=w811:T4)  [unwired: 5 in]
                n190 = call <vilib>:"Pack.vi"("Argument"=w788, "error in (no error)"=w807, "Python Object References In"=w809, "Session ID"=w811) -> ("error out"=w806:errorcluster, "Python Object References Out"=w802:T5, "Session ID out"=w798:T4)  [unwired: 5 in]
                n191 = call <vilib>:"Pack.vi"("Argument"=w787, "error in (no error)"=w806, "Python Object References In"=w802, "Session ID"=w798) -> ("error out"=w805:errorcluster, "Python Object References Out"=w801:T5, "Session ID out"=w797:T4)  [unwired: 5 in]
                n192 = call <vilib>:"Pack.vi"("Argument"="O2 frac 8", "error in (no error)"=w805, "Python Object References In"=w801, "Session ID"=w797) -> ("error out"=w804:errorcluster, "Python Object References Out"=w800:T5, "Session ID out"=w796:T4)  [unwired: 5 in]
                n193 = call <vilib>:"Pack.vi"("Argument"=w786, "error in (no error)"=w804, "Python Object References In"=w800, "Session ID"=w796) -> ("error out"=w803:errorcluster, "Python Object References Out"=w799:T5, "Session ID out"=w795:T4)  [unwired: 5 in]
                n194 = call <vilib>:"Call.vi"("Function or Method Name"="AppendResultFile", "error in (no error)"=w803, "Python Object References In"=w799, "Session ID"=w795) -> ("error out"=w822:errorcluster, "Session ID out"=w814:T4)  [unwired: 5 in, 1 out]
                n195 = call <vilib>:"Close Session.vi"("error in (no error)"=w822, "Session ID"=w814) -> ()  [unwired: 9 in, 1 out]
                "Temp 8" <- "Temp 8"
                "Flow 8" <- "Flow 8"
                "Conc 8" <- "Conc 8"
                "O2 frac 8" <- "O2 frac 8"
              }
            }
            "Exp 8" <- TRUE
          }
          frame 10 {
            n196 = flat-sequence {
              tunnel: w833 -> [w851]
              tunnel: w829 -> [w844]
              tunnel: w829 -> [_]
              tunnel: w829 -> [_]
              frame #0 {
                n197 = call <vilib>:"New Session.vi"("Path to Python Module (.py File)"=path "C:/Users/User/Documents/LabVIEW Data/2015 Projects/Combined/HMF_onlineHPLC.py") -> ("error out"=w861:errorcluster, "Session ID out"=w860:T4)  [unwired: 9 in]
                n198 = call <vilib>:"Pack.vi"("Argument"=w851, "error in (no error)"=w861, "Session ID"=w860) -> ("error out"=w850:errorcluster, "Python Object References Out"=w849:T5, "Session ID out"=w848:T4)  [unwired: 6 in]
                n199 = call <vilib>:"Pack.vi"("Argument"=w844, "error in (no error)"=w850, "Python Object References In"=w849, "Session ID"=w848) -> ("error out"=w845:errorcluster, "Python Object References Out"=w846:T5, "Session ID out"=w847:T4)  [unwired: 5 in]
                n200 = call <vilib>:"Call.vi"("Function or Method Name"="HPLC", "error in (no error)"=w845, "Python Object References In"=w846, "Session ID"=w847) -> ("error out"=w862:errorcluster, "Python Object References Out"=w854:T5, "Session ID out"=w855:T4)  [unwired: 5 in]
                n201 = call-poly <vilib>:"Unpack.vi"("error in (no error)"=w862, "Python Object References In"=w854, "Session ID"=w855) -> ("error out"=w863:errorcluster, "Value"=→"C HMF 8":dbl, "Python Object References Out"=w859:T5, "Session ID out"=w858:T4)  [unwired: 5 in]
                n202 = call-poly <vilib>:"Unpack.vi"("error in (no error)"=w863, "Python Object References In"=w859, "Session ID"=w858) -> ("error out"=w835:errorcluster, "Value"=→"C HFCA 8":dbl, "Python Object References Out"=w834:T5, "Session ID out"=w836:T4)  [unwired: 5 in]
                n203 = call-poly <vilib>:"Unpack.vi"("error in (no error)"=w835, "Python Object References In"=w834, "Session ID"=w836) -> ("error out"=w843:errorcluster, "Value"=→"C FFCA 8":dbl, "Python Object References Out"=w842:T5, "Session ID out"=w841:T4)  [unwired: 5 in]
                n204 = call-poly <vilib>:"Unpack.vi"("error in (no error)"=w843, "Python Object References In"=w842, "Session ID"=w841) -> ("error out"=w837:errorcluster, "Value"=→"C FDCA 8":dbl, "Session ID out"=w838:T4)  [unwired: 5 in, 1 out]
                n205 = call <vilib>:"Close Session.vi"("error in (no error)"=w837, "Session ID"=w838) -> ()  [unwired: 9 in, 1 out]
              }
              frame #1 {
              }
              frame #2 {
              }
            }
          }
        }
      }
      frame True {
        w866 = 0
      }
    }
    n206 = timed-loop {
      tunnel: w166 -> [w1050]
      tunnel: w165 -> [w1049]
      tunnel: [w998] -> w164
      tunnel: [w997] -> w163
      timing: w162 -> [_]
      timing-out: [_] -> w161
      tunnel: w160 -> [w984]
      tunnel: w159 -> [w988]
      tunnel: w158 -> [w987]
      tunnel: [w983] -> w157
      tunnel: [w982] -> w156
      tunnel: [w882] -> w155
      tunnel: w146 -> [w980]
      tunnel: w145 -> [w979]
      tunnel: w144 -> [w939]
      tunnel: w154 -> [w970]
      tunnel: w153 -> [w969]
      tunnel: w152 -> [w968]
      tunnel: w151 -> [w967]
      tunnel: [w965] -> w150
      tunnel: [w964] -> w149
      tunnel: ["Stop everything"] -> w147
      tunnel: "Automated Experiments or Direct Control" -> [w873]
      tunnel: w133 -> [w934]
      tunnel: w132 -> [w933]
      tunnel: [w932] -> w131
      tunnel: [w931] -> w130
      tunnel: w124 -> [w910]
      tunnel: w123 -> [w909]
      tunnel: w122 -> [w908]
      tunnel: w121 -> [w907]
      tunnel: w120 -> [w906]
      tunnel: w119 -> [w905]
      tunnel: w113 -> [w872]
      tunnel: w112 -> [w871]
      i -> [w958]
      stop <- w884 stop-if-true
      w924 = 0
      w923 = 0.1
      w904 = 7.5 ("Safety Shut Down Pressure (barg)")
      # "turn off gas if stop or if safety limit reached\nbut not for skip or end of exp"
      # "Emergency shut down, turns off gas"
      # "or stop"
      # "or change set point"
      # "or read sp"
      # "or test gas comm"
      # "pressure"
      # "syringe"
      # "temperature"
      # "Conc HMF in HMF Syringes"
      # "Conc HMF in NaOH Syringes"
      # "Any pressures"
      # "in case out of range changes conc to within possible range"
      # "1st 4 flowrates\n5,6 temperatures\n7 pressure (1)\n8 gas (1)"
      # "temperature or syringe or  pressure"
      # "We are graphing in barg"
      # "temperature or syringe"
      # "Empty Syringe has level of 50"
      n207 = node-c288() -> ()  [unwired: 1 in, 1 out]
      n208 = call-poly <vilib>:"DAQmx Read.vi"("task/channels in"=w934, "error in"=w933) -> ("task out"=w932:refnum<k21>, "data"=w927:dbl, "error out"=w931:errorcluster)  [unwired: 11 in]
      n209 = Multiply(x=5.1522, y=w927) -> (x*y=w930:dbl)
      n210 = Add(x=-2.6852, y=w930) -> (x+y=→"Liquid Inlet Pressure (bar g)":dbl)
      n211 = case shown="False" "Test Gas Communication" {
        frame False {
        }
        frame True {
          w1250 = "?BSI_Test"  # ?BSI_Test
          n212 = stacked-sequence {
            seq-local: [w1251 _ _] -> [_ _ w1284]
            tunnel: w1250 -> [w1251 _ _]
            frame #0 {
              # "Write Text to Clipboard"
              n213 = String Length(string=w1251) -> (length=w1260:i32)
              n214 = Increment(x=w1260) -> (x+1=w1256:i32)
              n215 = dll-call lib="kernel32" fn="GlobalAlloc"("Flags"=i16 0 ("Format"), "Size"=w1256) -> (w1255:i32)  [unwired: 5 in, 2 out]
              n216 = dll-call lib="kernel32" fn="GlobalLock"("hGlobalMemory"=w1255) -> (w1258:i32)  [unwired: 4 in, 2 out]
              n217 = dll-call lib="kernel32" fn="lstrcpy"("Flags"=w1258, "String"=w1251) -> (w1257:i32)  [unwired: 5 in, 2 out]
              n218 = stacked-sequence {
                tunnel: w1257 -> [_]
                tunnel: w1255 -> [w1279]
                tunnel: [w1278] -> w1254
                frame #0 {
                  n219 = dll-call lib="kernel32" fn="LocalUnlock"("hGlobalMemory"=w1279) -> (w1278:i32)  [unwired: 4 in, 2 out]
                }
              }
              "Error Out" <- w1254
              n220 = case shown="1, Default" w1254 {
                selector: w1254 -> [_ w1275]
                tunnel: w1255 -> [w1261 _]
                tunnel: [w1262 w1274] -> w1253
                frame 0 {
                  n221 = dll-call lib="user32" fn="OpenClipboard"("owner"=i16 0) -> (w1263:i32)  [unwired: 4 in, 2 out]
                  n222 = case shown="0" w1263 {
                    selector: w1263 -> [w1267 _]
                    tunnel: [w1265 w1270] -> w1262
                    tunnel: w1261 -> [_ w1269]
                    frame 0 {
                      n223 = Equal To 0?(x=w1267) -> (x = 0?=w1268:bool)
                      n224 = Bundle(w1268, w1267, "source"="Error opening clipboard") -> (w1265:cluster{bool, i32, "source":string})  [unwired: 1 in]
                    }
                    frame 1, Default {
                      n225 = stacked-sequence {
                        tunnel: [_ _ _ cluster{bool, i32, "source":string} {FALSE, 0, "source"=""} ("Output Element")] -> w1270
                        tunnel: w1269 -> [_ w1271 _ _]
                        frame #0 {
                          n226 = dll-call lib="user32" fn="EmptyClipboard"() -> ()  [unwired: 4 in, 2 out]
                        }
                        frame #1 {
                          n227 = dll-call lib="user32" fn="SetClipboardData"("Format"=1, "Data"=w1271) -> ()  [unwired: 6 in, 2 out]
                        }
                        frame #2 {
                          n228 = dll-call lib="user32" fn="CloseClipboard"() -> ()  [unwired: 4 in, 2 out]
                        }
                        frame #3 {
                        }
                      }
                    }
                  }
                }
                frame 1, Default {
                  n229 = Not Equal To 0?(x=w1275) -> (x != 0?=w1276:bool)
                  n230 = Bundle(w1276, w1275, "source"="Error copying text to clipboard") -> (w1274:cluster{bool, i32, "source":string})  [unwired: 1 in]
                }
              }
              "Write error out" <- w1253
              n231 = local write "Test Status"("Running" ("Status")) -> ()
            }
            frame #1 {
              # "Wait 500 milliseconds"
              n232 = Wait (ms)(milliseconds to wait=u32 500) -> ()  [unwired: 1 out]
            }
            frame #2 {
              # "Read Text From Clipboard"
              n233 = dll-call lib="user32" fn="OpenClipboard"("owner"=i16 0) -> (w1286:i32)  [unwired: 4 in, 2 out]
              n234 = case shown="1, Default" w1286 {
                selector: w1286 -> [w1292 _]
                tunnel: ["" w1297] -> w1281
                tunnel: [w1290 cluster{bool, i32, "source":string} {FALSE, 0, "source"=""} ("Output Element")] -> w1285
                frame 0 {
                  n235 = Equal To 0?(x=w1292) -> (x = 0?=w1293:bool)
                  n236 = Bundle(w1293, w1292, "source"="No text in clipboard available!") -> (w1290:cluster{bool, i32, "source":string})  [unwired: 1 in]
                }
                frame 1, Default {
                  n237 = dll-call lib="user32" fn="GetClipboardData"("uFormat"=1 ("hGlobalMemory")) -> (w1298:i32)  [unwired: 4 in, 2 out]
                  n238 = dll-call lib="kernel32" fn="GlobalLock"("hGlobalMemory"=w1298) -> (w1297:string, "hGlobalMemory"=w1295:i32)  [unwired: 3 in, 2 out]
                  n239 = stacked-sequence {
                    tunnel: w1295 -> [w1300 _]
                    frame #0 {
                      n240 = dll-call lib="kernel32" fn="LocalUnlock"("hGlobalMemory"=w1300) -> ()  [unwired: 5 in, 2 out]
                    }
                    frame #1 {
                      n241 = dll-call lib="user32" fn="CloseClipboard"() -> ()  [unwired: 4 in, 2 out]
                    }
                  }
                }
              }
              "Text Read From Clipboard" <- w1281
              "Read error out" <- w1285
              n242 = Equal?(x=w1284, y=w1281) -> (x = y?=w1283:bool)
              n243 = case shown="True" w1283 {
                tunnel: ["Response OK" "Failed: No Response from Lab Interface"] -> w1282
                frame False {
                }
                frame True {
                }
              }
              "Test Status" <- w1282
            }
          }
        }
      }
      n244 = case shown="False" "Read Set Points" {
        frame False {
        }
        frame True {
          w1199 = "?BSI_ReadFlowSetPoints"  # ?BSI_ReadFlowSetPoints
          n245 = stacked-sequence {
            seq-local: [w1200 _ _] -> [_ _ w1233]
            tunnel: w1199 -> [w1200 _ _]
            frame #0 {
              # "Write Text to Clipboard"
              n246 = String Length(string=w1200) -> (length=w1209:i32)
              n247 = Increment(x=w1209) -> (x+1=w1205:i32)
              n248 = dll-call lib="kernel32" fn="GlobalAlloc"("Flags"=i16 0 ("Format"), "Size"=w1205) -> (w1204:i32)  [unwired: 5 in, 2 out]
              n249 = dll-call lib="kernel32" fn="GlobalLock"("hGlobalMemory"=w1204) -> (w1207:i32)  [unwired: 4 in, 2 out]
              n250 = dll-call lib="kernel32" fn="lstrcpy"("Flags"=w1207, "String"=w1200) -> (w1206:i32)  [unwired: 5 in, 2 out]
              n251 = stacked-sequence {
                tunnel: w1206 -> [_]
                tunnel: w1204 -> [w1228]
                tunnel: [w1227] -> w1203
                frame #0 {
                  n252 = dll-call lib="kernel32" fn="LocalUnlock"("hGlobalMemory"=w1228) -> (w1227:i32)  [unwired: 4 in, 2 out]
                }
              }
              "Error Out 3" <- w1203
              n253 = case shown="0" w1203 {
                selector: w1203 -> [_ w1224]
                tunnel: w1204 -> [w1210 _]
                tunnel: [w1211 w1223] -> w1202
                frame 0 {
                  n254 = dll-call lib="user32" fn="OpenClipboard"("owner"=i16 0) -> (w1212:i32)  [unwired: 4 in, 2 out]
                  n255 = case shown="1, Default" w1212 {
                    selector: w1212 -> [w1216 _]
                    tunnel: [w1214 w1219] -> w1211
                    tunnel: w1210 -> [_ w1218]
                    frame 0 {
                      n256 = Equal To 0?(x=w1216) -> (x = 0?=w1217:bool)
                      n257 = Bundle(w1217, w1216, "source"="Error opening clipboard") -> (w1214:cluster{bool, i32, "source":string})  [unwired: 1 in]
                    }
                    frame 1, Default {
                      n258 = stacked-sequence {
                        tunnel: [_ _ _ cluster{bool, i32, "source":string} {FALSE, 0, "source"=""} ("Output Element")] -> w1219
                        tunnel: w1218 -> [_ w1220 _ _]
                        frame #0 {
                          n259 = dll-call lib="user32" fn="EmptyClipboard"() -> ()  [unwired: 4 in, 2 out]
                        }
                        frame #1 {
                          n260 = dll-call lib="user32" fn="SetClipboardData"("Format"=1, "Data"=w1220) -> ()  [unwired: 6 in, 2 out]
                        }
                        frame #2 {
                          n261 = dll-call lib="user32" fn="CloseClipboard"() -> ()  [unwired: 4 in, 2 out]
                        }
                        frame #3 {
                        }
                      }
                    }
                  }
                }
                frame 1, Default {
                  n262 = Not Equal To 0?(x=w1224) -> (x != 0?=w1225:bool)
                  n263 = Bundle(w1225, w1224, "source"="Error copying text to clipboard") -> (w1223:cluster{bool, i32, "source":string})  [unwired: 1 in]
                }
              }
              "Write error out 3" <- w1202
              n264 = local write "Read Set Point Status"("Running" ("Status")) -> ()
            }
            frame #1 {
              # "Wait 500 milliseconds"
              n265 = Wait (ms)(milliseconds to wait=u32 500) -> ()  [unwired: 1 out]
            }
            frame #2 {
              # "Read Text From Clipboard"
              n266 = dll-call lib="user32" fn="OpenClipboard"("owner"=i16 0) -> (w1235:i32)  [unwired: 4 in, 2 out]
              n267 = case shown="1, Default" w1235 {
                selector: w1235 -> [w1241 _]
                tunnel: ["" w1246] -> w1230
                tunnel: [w1239 cluster{bool, i32, "source":string} {FALSE, 0, "source"=""} ("Output Element")] -> w1234
                frame 0 {
                  n268 = Equal To 0?(x=w1241) -> (x = 0?=w1242:bool)
                  n269 = Bundle(w1242, w1241, "source"="No text in clipboard available!") -> (w1239:cluster{bool, i32, "source":string})  [unwired: 1 in]
                }
                frame 1, Default {
                  n270 = dll-call lib="user32" fn="GetClipboardData"("uFormat"=1 ("hGlobalMemory")) -> (w1247:i32)  [unwired: 4 in, 2 out]
                  n271 = dll-call lib="kernel32" fn="GlobalLock"("hGlobalMemory"=w1247) -> (w1246:string, "hGlobalMemory"=w1244:i32)  [unwired: 3 in, 2 out]
                  n272 = stacked-sequence {
                    tunnel: w1244 -> [w1249 _]
                    frame #0 {
                      n273 = dll-call lib="kernel32" fn="LocalUnlock"("hGlobalMemory"=w1249) -> ()  [unwired: 5 in, 2 out]
                    }
                    frame #1 {
                      n274 = dll-call lib="user32" fn="CloseClipboard"() -> ()  [unwired: 4 in, 2 out]
                    }
                  }
                }
              }
              "Text Read From Clipboard 3" <- w1230
              "Read error out 3" <- w1234
              n275 = Equal?(x=w1233, y=w1230) -> (x = y?=w1232:bool)
              n276 = case shown="True" w1232 {
                tunnel: ["Response OK" "Failed: No Response from Lab Interface"] -> w1231
                frame False {
                }
                frame True {
                }
              }
              "Read Set Point Status" <- w1231
            }
          }
        }
      }
      n277 = for {
        N: 4 -> [_]
        tunnel: w1050 -> [w1663] mode=indexing
        tunnel: [w1661] -> w1044 mode=indexing
        tunnel: [w1658] -> w1039 mode=indexing
        tunnel: [w1657] -> w1038 mode=indexing
        tunnel: [w1656] -> w1037 mode=indexing
        tunnel: w1049 -> [w1655] mode=indexing
        i -> [w1662]
        n278 = call "NCS_GetFlowRateIs.vi"("error in (no error)"=w1655, "dosingunit"=w1662, "device handle in"=w1663) -> ("error out"=w1659:errorcluster, "flowrate is"=w1661:dbl, "device handle out"=w1660:u32)
        n279 = call "NCS_GetSyringeLevelIs.vi"("error in (no error)"=w1659, "dosingunit"=w1662, "device handle in"=w1660) -> ("error out"=w1656:errorcluster, "syringe level is"=w1658:dbl, "device handle out"=w1657:u32)
      }
      n280 = Index Array(array=w1039, index=0) -> (element=w962:dbl)
      "Syringe Level 1" <- w962
      n281 = Index Array(array=w1039, index=3) -> (element=w959:dbl)
      "Syringe Level 4" <- w959
      n282 = Index Array(array=w1039, index=1) -> (element=w961:dbl)
      "Syringe Level 2" <- w961
      n283 = Index Array(array=w1039, index=2) -> (element=w960:dbl)
      "Syringe Level 3" <- w960
      n284 = case shown="True" "Shut down in empty?\nLeft off, right on" {
        tunnel: [FALSE w1549] -> w868
        tunnel: w962 -> [_ w1548]
        tunnel: w961 -> [_ w1547]
        tunnel: w960 -> [_ w1546]
        tunnel: w959 -> [_ w1545]
        frame False {
        }
        frame True {
          w1550 = 75
          n285 = Less Or Equal?(x=w1547, y=w1550) -> (x <= y?=w1556:bool)
          n286 = Less Or Equal?(x=w1548, y=w1550) -> (x <= y?=w1551:bool)
          n287 = Less Or Equal?(x=w1546, y=w1550) -> (x <= y?=w1554:bool)
          n288 = Less Or Equal?(x=w1545, y=w1550) -> (x <= y?=w1552:bool)
          n289 = Or(x=w1551, y=w1556) -> (x .or. y?=w1555:bool)
          n290 = Or(x=w1555, y=w1554) -> (x .or. y?=w1553:bool)
          n291 = Or(x=w1553, y=w1552) -> (x .or. y?=w1549:bool)
        }
      }
      "syringe limit empty" <- w868
      n292 = Index Array(array=w1044, index=0) -> (element=w948:dbl)
      "Flowrate 1 HMF" <- w948
      n293 = Index Array(array=w1044, index=3) -> (element=w950:dbl)
      "Flowrate 4 NaOH" <- w950
      n294 = Index Array(array=w1044, index=1) -> (element=w947:dbl)
      "Flowrate 2 NaOH or HMF" <- w947
      n295 = Index Array(array=w1044, index=2) -> (element=w925:dbl)
      "Flowrate 3 NaOH" <- w925
      n296 = call-poly <vilib>:"DAQmx Read.vi"("task/channels in"=w970, "error in"=w969) -> ("task out"=w965:refnum<k21>, "data"=w892:dbl[], "error out"=w964:errorcluster)  [unwired: 11 in]
      n297 = Add(x=w948, y=w947) -> (x+y=w952:dbl)
      n298 = Add(x=w952, y=w925) -> (x+y=w951:dbl)
      n299 = Index Array(array=w892, index=3) -> (element=w890:dbl)
      n300 = Index Array(array=w892, index=2) -> (element=w891:dbl)
      n301 = Index Array(array=w892, index=1) -> (element=w893:dbl)
      n302 = Index Array(array=w892, index=0) -> (element=w973:dbl)
      n303 = Add(x=w951, y=w950) -> (x+y=w949:dbl)
      "Total Flowrate (uL/min)" <- w949
      n304 = Divide(x=w948, y=w949) -> (x/y=w942:dbl)
      n305 = Multiply(x=w890, y=w906) -> (x*y=w913:dbl)
      n306 = Multiply(x=w891, y=w908) -> (x*y=w917:dbl)
      n307 = Multiply(x=w893, y=w910) -> (x*y=w921:dbl)
      n308 = Multiply(x=w973, y=w968) -> (x*y=w974:dbl)
      n309 = Multiply(x=w924, y=w942) -> (x*y=w946:dbl)
      n310 = Add(x=w913, y=w905) -> (x+y=w911:dbl)
      n311 = Add(x=w917, y=w907) -> (x+y=w915:dbl)
      n312 = Add(x=w921, y=w909) -> (x+y=w919:dbl)
      n313 = Divide(x=w925, y=w949) -> (x/y=w943:dbl)
      n314 = Add(x=w974, y=w967) -> (x+y=w971:dbl)
      n315 = Multiply(x=w923, y=w943) -> (x*y=w945:dbl)
      n316 = Add(x=w946, y=w945) -> (x+y=→"Feed Concentration if 2 syringe (M)":dbl)
      n317 = In Range and Coerce(upper limit=w923, x=w939, lower limit=w924) -> (coerced(x)=w936:dbl, In Range?=w938:bool)
      n318 = case shown="True" w938 {
        tunnel: [w1381 w1383] -> w937
        tunnel: w939 -> [_ w1383]
        tunnel: w936 -> [w1381 _]
        tunnel: [TRUE FALSE] -> w935
        frame False {
        }
        frame True {
        }
      }
      "Desired Conc Not Possible" <- w935
      n319 = Multiply(x=w911, y=0.0689476) -> (x*y=w900:dbl)
      "Nitrogen Pressure (barg)" <- w900
      n320 = Multiply(x=w915, y=0.0689476) -> (x*y=w901:dbl)
      "Reactor Gas Back Pressure (barg)" <- w901
      n321 = Multiply(x=w919, y=0.0689476) -> (x*y=w902:dbl)
      "Nitrogen Gas  Pressure (barg)" <- w902
      n322 = Multiply(x=w971, y=0.0689476) -> (x*y=w903:dbl)
      "Oxygen Gas Pressure (barg)" <- w903
      n323 = case shown="False" w873 {
        tunnel: [w1618 w1636] -> w1035
        tunnel: w979 -> [w1614 _]
        tunnel: w937 -> [w1616 _]
        tunnel: w923 -> [w1617 _]
        tunnel: w924 -> [w1615 _]
        frame False {
          # "h-s/h-l"
          # "s-l/h-l"
          # "high flow"
          # "low flow"
          # "Number of Syringes"
          # "h-s"
          # "s-l"
          # "h-l"
          n324 = case shown="False" "2 Syringes or 4 Syringes" {
            tunnel: [1 2] -> w1613
            frame False {
            }
            frame True {
            }
          }
          n325 = Subtract(x=w1617, y=w1615) -> (x-y=w1619:dbl)
          n326 = Subtract(x=w1616, y=w1615) -> (x-y=w1624:dbl)
          n327 = Subtract(x=w1617, y=w1616) -> (x-y=w1620:dbl)
          n328 = Divide(x=w1614, y=w1613) -> (x/y=w1623:dbl)
          n329 = Divide(x=w1620, y=w1619) -> (x/y=w1622:dbl)
          n330 = Divide(x=w1624, y=w1619) -> (x/y=w1621:dbl)
          n331 = Multiply(x=w1623, y=w1622) -> (x*y=w1612:dbl)
          n332 = Multiply(x=w1623, y=w1621) -> (x*y=w1611:dbl)
          n333 = case shown="False" "2 Syringes or 4 Syringes" {
            tunnel: [w1631 w1633] -> w1610
            tunnel: w1612 -> [w1631 w1633]
            tunnel: [w1629 w1632] -> w1609
            tunnel: w1611 -> [w1630 w1632]
            tunnel: [w1630 w1633] -> w1605
            tunnel: [w1629 w1632] -> w1604
            frame False {
              w1629 = 0
            }
            frame True {
            }
          }
          n334 = case shown="False" "NaOH in 3 or NaOH in 2" {
            tunnel: [w1625 w1628] -> w1606
            tunnel: w1605 -> [w1626 w1628]
            tunnel: [w1626 w1627] -> w1603
            tunnel: w1604 -> [w1625 w1627]
            frame False {
              # "NaOH in 3"
            }
            frame True {
              # "naOH in 2"
            }
          }
          n335 = Build Array(w1610, w1606, w1603, w1609) -> (w1618:dbl[])
        }
        frame True {
          n336 = Build Array("Set Flowrate 1", "Set Flowrate 2", "Set Flowrate 3", "Set Flowrate 4") -> (w1636:dbl[])
        }
      }
      n337 = Greater Or Equal?(x=w902, y=w904) -> (x >= y?=w898:bool)
      n338 = Greater Or Equal?(x=w903, y=w904) -> (x >= y?=w899:bool)
      n339 = Greater Or Equal?(x=w901, y=w904) -> (x >= y?=w896:bool)
      n340 = Greater Or Equal?(x=w900, y=w904) -> (x >= y?=w894:bool)
      n341 = Or(x=w899, y=w898) -> (x .or. y?=w897:bool)
      n342 = Or(x=w897, y=w896) -> (x .or. y?=w895:bool)
      n343 = Or(x=w895, y=w894) -> (x .or. y?=w869:bool)
      "Pressure limit reached" <- w869
      n344 = case shown="False" w873 {
        tunnel: [w1558 FALSE] -> w874
        tunnel: w958 -> [w1557 _]
        frame False {
          # "changes set points for each new exp"
          n345 = Equal?(x=w1557, y=0) -> (x = y?=w1558:bool)
        }
        frame True {
          # "at end of each exp"
          # "doesnt automatically change set point"
        }
      }
      n346 = Or(x=w874, y="Change New Set Points") -> (x .or. y?=w875:bool)
      n347 = Or(x="Read Set Points", y=w875) -> (x .or. y?=w887:bool)
      n348 = case shown="True" w875 {
        tunnel: w873 -> [_ w1121]
        tunnel: w872 -> [_ w1120]
        tunnel: w871 -> [_ w1119]
        frame False {
        }
        frame True {
          w1107 = 1
          w1116 = 1.1112
          w1110 = 1.1159
          w1113 = 1.1444
          w1142 = 20
          w1135 = ","
          n349 = case shown="False" w1121 {
            tunnel: [w1145 "Set Point 2 (NmL/min)"] -> w1114
            tunnel: [w1146 "Set Point 1 (NmL/min)"] -> w1117
            tunnel: w1120 -> [w1144 _]
            tunnel: w1119 -> [w1143 _]
            frame False {
              n350 = Multiply(x=w1144, y=w1143) -> (x*y=w1146:dbl)
              n351 = Subtract(x=w1143, y=w1146) -> (x-y=w1145:dbl)
            }
            frame True {
            }
          }
          n352 = Divide(x="Set Point 4 (NmL/min)", y=w1107) -> (x/y=w1108:dbl)
          n353 = Divide(x="Set Point 3 (NmL/min)", y=w1110) -> (x/y=w1111:dbl)
          n354 = Divide(x=w1114, y=w1113) -> (x/y=w1115:dbl)
          n355 = Divide(x=w1117, y=w1116) -> (x/y=w1118:dbl)
          n356 = Divide(x=w1118, y=w1142) -> (x/y=w1122:dbl)
          n357 = Divide(x=w1115, y=w1142) -> (x/y=w1124:dbl)
          n358 = Divide(x=w1111, y=w1142) -> (x/y=w1126:dbl)
          n359 = Divide(x=w1108, y=w1142) -> (x/y=w1128:dbl)
          n360 = Multiply(x=w1122, y=100) -> (x*y=w1130:dbl)
          n361 = Multiply(x=w1124, y=100) -> (x*y=w1131:dbl)
          n362 = Multiply(x=w1126, y=100) -> (x*y=w1132:dbl)
          n363 = Multiply(x=w1128, y=100) -> (x*y=w1133:dbl)
          n364 = Format Into String(w1131) -> (resulting string=w1138:string)  [unwired: 3 in, 1 out]
          n365 = Format Into String(w1130) -> (resulting string=w1137:string)  [unwired: 3 in, 1 out]
          n366 = Format Into String(w1132) -> (resulting string=w1139:string)  [unwired: 3 in, 1 out]
          n367 = Format Into String(w1133) -> (resulting string=w1140:string)  [unwired: 3 in, 1 out]
          n368 = Concatenate Strings("?BSI_SetFlowSetPoints ", w1137, w1135, w1138, w1135, w1139, w1135, w1140, w1135, "*,*,*,*,*,*,*,*,*,*,*,*,*,*,*,*,*,*,*,*,*,*,*,*,*,*") -> (w1141:string)
          "Set Point Function" <- w1141
          n369 = stacked-sequence {
            seq-local: [w1149 _ _] -> [_ _ w1182]
            tunnel: w1141 -> [w1149 _ _]
            frame #0 {
              # "Write Text to Clipboard"
              n370 = String Length(string=w1149) -> (length=w1158:i32)
              n371 = Increment(x=w1158) -> (x+1=w1154:i32)
              n372 = dll-call lib="kernel32" fn="GlobalAlloc"("Flags"=i16 0 ("Format"), "Size"=w1154) -> (w1153:i32)  [unwired: 5 in, 2 out]
              n373 = dll-call lib="kernel32" fn="GlobalLock"("hGlobalMemory"=w1153) -> (w1156:i32)  [unwired: 4 in, 2 out]
              n374 = dll-call lib="kernel32" fn="lstrcpy"("Flags"=w1156, "String"=w1149) -> (w1155:i32)  [unwired: 5 in, 2 out]
              n375 = stacked-sequence {
                tunnel: w1155 -> [_]
                tunnel: w1153 -> [w1177]
                tunnel: [w1176] -> w1152
                frame #0 {
                  n376 = dll-call lib="kernel32" fn="LocalUnlock"("hGlobalMemory"=w1177) -> (w1176:i32)  [unwired: 4 in, 2 out]
                }
              }
              "Error Out 4" <- w1152
              n377 = case shown="0" w1152 {
                selector: w1152 -> [_ w1173]
                tunnel: w1153 -> [w1159 _]
                tunnel: [w1160 w1172] -> w1151
                frame 0 {
                  n378 = dll-call lib="user32" fn="OpenClipboard"("owner"=i16 0) -> (w1161:i32)  [unwired: 4 in, 2 out]
                  n379 = case shown="1, Default" w1161 {
                    selector: w1161 -> [w1165 _]
                    tunnel: [w1163 w1168] -> w1160
                    tunnel: w1159 -> [_ w1167]
                    frame 0 {
                      n380 = Equal To 0?(x=w1165) -> (x = 0?=w1166:bool)
                      n381 = Bundle(w1166, w1165, "source"="Error opening clipboard") -> (w1163:cluster{bool, i32, "source":string})  [unwired: 1 in]
                    }
                    frame 1, Default {
                      n382 = stacked-sequence {
                        tunnel: [_ _ _ cluster{bool, i32, "source":string} {FALSE, 0, "source"=""} ("Output Element")] -> w1168
                        tunnel: w1167 -> [_ w1169 _ _]
                        frame #0 {
                          n383 = dll-call lib="user32" fn="EmptyClipboard"() -> ()  [unwired: 4 in, 2 out]
                        }
                        frame #1 {
                          n384 = dll-call lib="user32" fn="SetClipboardData"("Format"=1, "Data"=w1169) -> ()  [unwired: 6 in, 2 out]
                        }
                        frame #2 {
                          n385 = dll-call lib="user32" fn="CloseClipboard"() -> ()  [unwired: 4 in, 2 out]
                        }
                        frame #3 {
                        }
                      }
                    }
                  }
                }
                frame 1, Default {
                  n386 = Not Equal To 0?(x=w1173) -> (x != 0?=w1174:bool)
                  n387 = Bundle(w1174, w1173, "source"="Error copying text to clipboard") -> (w1172:cluster{bool, i32, "source":string})  [unwired: 1 in]
                }
              }
              "Write error out 4" <- w1151
              n388 = local write "Write Set Point Status"("Running" ("Status")) -> ()
            }
            frame #1 {
              # "Wait 500 milliseconds"
              n389 = Wait (ms)(milliseconds to wait=u32 500) -> ()  [unwired: 1 out]
            }
            frame #2 {
              # "Read Text From Clipboard"
              n390 = dll-call lib="user32" fn="OpenClipboard"("owner"=i16 0) -> (w1184:i32)  [unwired: 4 in, 2 out]
              n391 = case shown="1, Default" w1184 {
                selector: w1184 -> [w1190 _]
                tunnel: ["" w1195] -> w1179
                tunnel: [w1188 cluster{bool, i32, "source":string} {FALSE, 0, "source"=""} ("Output Element")] -> w1183
                frame 0 {
                  n392 = Equal To 0?(x=w1190) -> (x = 0?=w1191:bool)
                  n393 = Bundle(w1191, w1190, "source"="No text in clipboard available!") -> (w1188:cluster{bool, i32, "source":string})  [unwired: 1 in]
                }
                frame 1, Default {
                  n394 = dll-call lib="user32" fn="GetClipboardData"("uFormat"=1 ("hGlobalMemory")) -> (w1196:i32)  [unwired: 4 in, 2 out]
                  n395 = dll-call lib="kernel32" fn="GlobalLock"("hGlobalMemory"=w1196) -> (w1195:string, "hGlobalMemory"=w1193:i32)  [unwired: 3 in, 2 out]
                  n396 = stacked-sequence {
                    tunnel: w1193 -> [w1198 _]
                    frame #0 {
                      n397 = dll-call lib="kernel32" fn="LocalUnlock"("hGlobalMemory"=w1198) -> ()  [unwired: 5 in, 2 out]
                    }
                    frame #1 {
                      n398 = dll-call lib="user32" fn="CloseClipboard"() -> ()  [unwired: 4 in, 2 out]
                    }
                  }
                }
              }
              "Text Read From Clipboard 4" <- w1179
              "Read error out 4" <- w1183
              n399 = Equal?(x=w1182, y=w1179) -> (x = y?=w1181:bool)
              n400 = case shown="True" w1181 {
                tunnel: ["Response OK" "Failed: No Response from Lab Interface"] -> w1180
                frame False {
                }
                frame True {
                }
              }
              "Write Set Point Status" <- w1180
            }
          }
          "Flow Span of All Controlers (NmL/min)" <- w1142
          "O2 Cal 1" <- w1116
          "N2 Cal 2" <- w1113
          "N2 Cal 3" <- w1110
          "N2 Cal 4" <- w1107
        }
      }
      n401 = Or(x=w887, y="Test Gas Communication") -> (x .or. y?=w888:bool)
      n402 = Or(x=w874, y="Update Temperature Set Point") -> (x .or. y?=w990:bool)
      n403 = case shown="True" w990 {
        tunnel: w988 -> [w1562 w1570]
        tunnel: w987 -> [w1561 w1569]
        tunnel: [w1562 w1568] -> w986
        tunnel: [w1561 w1567] -> w985
        tunnel: w984 -> [_ w1566]
        tunnel: w873 -> [_ w1564]
        tunnel: w980 -> [_ w1563]
        frame False {
        }
        frame True {
          n404 = case shown="False" w1564 {
            tunnel: [w1571 "Set Point (oC)"] -> w1565
            tunnel: w1563 -> [w1571 _]
            frame False {
            }
            frame True {
            }
          }
          n405 = call "CN7500_Write Set Point Value.vi"("Target Set Point Value"=w1565, "error in (no error)"=w1569, "Controller Number"=w1566, "VISA In"=w1570) -> ("error out"=w1567:errorcluster, "VISA Out"=w1568:refnum<visa-resource-name>)  [unwired: 6 in]
        }
      }
      n406 = Or(x="Generate Flow", y=w874) -> (x .or. y?=w941:bool)
      n407 = case shown="True" w941 {
        tunnel: w1038 -> [w1642 w1647]
        tunnel: w1037 -> [w1641 w1646]
        tunnel: [w1641 w1645] -> w954
        tunnel: [w1642 w1644] -> w953
        tunnel: w1035 -> [_ w1643]
        frame False {
        }
        frame True {
          n408 = for {
            N: 4 -> [_]
            tunnel: w1647 -> [w1654] mode=indexing
            tunnel: w1646 -> [w1653] mode=indexing
            tunnel: [w1652] -> w1645 mode=indexing
            tunnel: [w1651] -> w1644 mode=indexing
            tunnel: w1643 -> [w1649] mode=indexing
            i -> [w1650]
            n409 = call "NCS_GenerateFlow.vi"("error in (no error)"=w1653, "flowrate"=w1649, "dosingunit"=w1650, "device handle in"=w1654) -> ("error out"=w1652:errorcluster, "device handle out"=w1651:u32)
          }
        }
      }
      n410 = call "CN7500_Read Process Value.vi"("error in (no error)"=w985, "Controller Number"=w984, "VISA In"=w986) -> ("error out"=w983:errorcluster, "Set Point Value"=w976:dbl, "Process Value"=w977:dbl, "VISA Out"=w982:refnum<visa-resource-name>)  [unwired: 5 in]
      "Temp Set Point (oC)" <- w976
      "Actual Temp (oC)" <- w977
      n411 = Merge Signals(w977, w976) -> (→"Temperature":dynamicdata)
      n412 = case shown="False" "Temp  Limit OFF or ON" {
        tunnel: w977 -> [_ w1054]
        tunnel: [FALSE w1053] -> w870
        frame False {
        }
        frame True {
          w1055 = 180
          n413 = Greater Or Equal?(x=w1054, y=w1055) -> (x >= y?=w1053:bool)
          "Safety Shut Down Temp" <- w1055
        }
      }
      "Temp limit reached" <- w870
      n414 = Index Array(array=w954, index=0) -> (element=w1025:errorcluster)
      n415 = Index Array(array=w953, index=0) -> (element=w1026:u32)
      n416 = Index Array(array=w954, index=1) -> (element=w1019:errorcluster)
      n417 = Index Array(array=w953, index=1) -> (element=w1020:u32)
      n418 = case shown="False" "Stop Dose 2" {
        tunnel: w1020 -> [w1590 w1595]
        tunnel: w1019 -> [w1589 w1594]
        tunnel: [w1590 w1593] -> w1012
        tunnel: [w1589 w1592] -> w1011
        frame False {
        }
        frame True {
          n419 = call "NCS_Stop.vi"("error in (no error)"=w1594, "dosingunit"=1, "device handle in"=w1595) -> ("error out"=w1592:errorcluster, "device handle out"=w1593:u32)
        }
      }
      n420 = case shown="False" "Stop Dose 1" {
        tunnel: w1026 -> [w1597 w1602]
        tunnel: w1025 -> [w1596 w1601]
        tunnel: [w1597 w1600] -> w1014
        tunnel: [w1596 w1599] -> w1013
        frame False {
        }
        frame True {
          n421 = call "NCS_Stop.vi"("error in (no error)"=w1601, "dosingunit"=0, "device handle in"=w1602) -> ("error out"=w1599:errorcluster, "device handle out"=w1600:u32)
        }
      }
      n422 = Index Array(array=w954, index=3) -> (element=w1015:errorcluster)
      n423 = Index Array(array=w954, index=2) -> (element=w1017:errorcluster)
      n424 = Index Array(array=w953, index=3) -> (element=w1016:u32)
      n425 = Index Array(array=w953, index=2) -> (element=w1018:u32)
      n426 = case shown="False" "Stop Dose 3" {
        tunnel: w1018 -> [w1583 w1588]
        tunnel: w1017 -> [w1582 w1587]
        tunnel: [w1583 w1586] -> w1010
        tunnel: [w1582 w1585] -> w1009
        frame False {
        }
        frame True {
          n427 = call "NCS_Stop.vi"("error in (no error)"=w1587, "dosingunit"=2, "device handle in"=w1588) -> ("error out"=w1585:errorcluster, "device handle out"=w1586:u32)
        }
      }
      n428 = case shown="False" "Stop Dose 4" {
        tunnel: w1016 -> [w1576 w1581]
        tunnel: w1015 -> [w1575 w1580]
        tunnel: [w1576 w1579] -> w1008
        tunnel: [w1575 w1578] -> w1007
        frame False {
        }
        frame True {
          n429 = call "NCS_Stop.vi"("error in (no error)"=w1580, "dosingunit"=3, "device handle in"=w1581) -> ("error out"=w1578:errorcluster, "device handle out"=w1579:u32)
        }
      }
      n430 = case shown="False" "Safety or Emergency Syringe Control" {
        tunnel: w1014 -> [w1391 w1432]
        tunnel: w1013 -> [w1387 w1431]
        tunnel: w1012 -> [w1390 w1430]
        tunnel: w1011 -> [w1386 w1429]
        tunnel: w1010 -> [w1389 w1428]
        tunnel: w1009 -> [w1385 w1427]
        tunnel: w1008 -> [w1388 w1426]
        tunnel: w1007 -> [w1384 w1425]
        tunnel: [w1391 w1402] -> w1006
        tunnel: [w1390 w1401] -> w1005
        tunnel: [w1389 w1400] -> w1004
        tunnel: [w1388 w1399] -> w1003
        tunnel: [w1386 w1398] -> w1002
        tunnel: [w1385 w1397] -> w1001
        tunnel: [w1384 w1396] -> w1000
        tunnel: [w1387 w1392] -> w999
        frame False {
        }
        frame True {
          n431 = case shown="False" "Calibrate 2" {
            tunnel: w1430 -> [w1531 w1536]
            tunnel: w1429 -> [w1530 w1535]
            tunnel: [w1531 w1534] -> w1419
            tunnel: [w1530 w1533] -> w1418
            frame False {
            }
            frame True {
              n432 = call "NCS_Calibrate.vi"("error in (no error)"=w1535, "dosingunit"=1, "device handle in"=w1536) -> ("error out"=w1533:errorcluster, "device handle out"=w1534:u32)
            }
          }
          n433 = case shown="False" "Calibrate 3" {
            tunnel: w1428 -> [w1524 w1529]
            tunnel: w1427 -> [w1523 w1528]
            tunnel: [w1524 w1527] -> w1417
            tunnel: [w1523 w1526] -> w1416
            frame False {
            }
            frame True {
              n434 = call "NCS_Calibrate.vi"("error in (no error)"=w1528, "dosingunit"=2, "device handle in"=w1529) -> ("error out"=w1526:errorcluster, "device handle out"=w1527:u32)
            }
          }
          n435 = case shown="False" "Calibrate 1" {
            tunnel: w1432 -> [w1538 w1543]
            tunnel: w1431 -> [w1537 w1542]
            tunnel: [w1538 w1541] -> w1421
            tunnel: [w1537 w1540] -> w1420
            frame False {
            }
            frame True {
              n436 = call "NCS_Calibrate.vi"("error in (no error)"=w1542, "dosingunit"=0, "device handle in"=w1543) -> ("error out"=w1540:errorcluster, "device handle out"=w1541:u32)
            }
          }
          n437 = case shown="False" "Calibrate 4" {
            tunnel: w1426 -> [w1517 w1522]
            tunnel: w1425 -> [w1516 w1521]
            tunnel: [w1517 w1520] -> w1415
            tunnel: [w1516 w1519] -> w1414
            frame False {
            }
            frame True {
              n438 = call "NCS_Calibrate.vi"("error in (no error)"=w1521, "dosingunit"=3, "device handle in"=w1522) -> ("error out"=w1519:errorcluster, "device handle out"=w1520:u32)
            }
          }
          n439 = case shown="False" "Empty 2" {
            tunnel: w1419 -> [w1497 w1501]
            tunnel: w1418 -> [w1496 w1499]
            tunnel: [w1497 w1500] -> w1405
            tunnel: [w1496 w1498] -> w1406
            frame False {
            }
            frame True {
              w1503 = 1
              n440 = call "NCS_GetFlowRateMax.vi"("error in (no error)"=w1499, "dosingunit"=w1503, "device handle in"=w1501) -> ("error out"=w1504:errorcluster, "flow rate max"=w1502:dbl, "device handle out"=w1505:u32)
              n441 = call "NCS_EmptySyrige.vi"("error in (no error)"=w1504, "flowrate"=w1502, "dosingunit"=w1503, "device handle in"=w1505) -> ("error out"=w1498:errorcluster, "device handle out"=w1500:u32)
            }
          }
          n442 = case shown="False" "Empty 1" {
            tunnel: w1421 -> [w1507 w1515]
            tunnel: w1420 -> [w1506 w1512]
            tunnel: [w1507 w1513] -> w1403
            tunnel: [w1506 w1510] -> w1404
            frame False {
            }
            frame True {
              w1509 = 0
              n443 = call "NCS_GetFlowRateMax.vi"("error in (no error)"=w1512, "dosingunit"=w1509, "device handle in"=w1515) -> ("error out"=w1511:errorcluster, "flow rate max"=w1508:dbl, "device handle out"=w1514:u32)
              n444 = call "NCS_EmptySyrige.vi"("error in (no error)"=w1511, "flowrate"=w1508, "dosingunit"=w1509, "device handle in"=w1514) -> ("error out"=w1510:errorcluster, "device handle out"=w1513:u32)
            }
          }
          n445 = case shown="False" "Empty 3" {
            tunnel: w1417 -> [w1487 w1488]
            tunnel: w1416 -> [w1486 w1489]
            tunnel: [w1487 w1490] -> w1407
            tunnel: [w1486 w1491] -> w1408
            frame False {
            }
            frame True {
              w1493 = 2
              n446 = call "NCS_GetFlowRateMax.vi"("error in (no error)"=w1489, "dosingunit"=w1493, "device handle in"=w1488) -> ("error out"=w1494:errorcluster, "flow rate max"=w1492:dbl, "device handle out"=w1495:u32)
              n447 = call "NCS_EmptySyrige.vi"("error in (no error)"=w1494, "flowrate"=w1492, "dosingunit"=w1493, "device handle in"=w1495) -> ("error out"=w1491:errorcluster, "device handle out"=w1490:u32)
            }
          }
          n448 = case shown="False" "Empty 4" {
            tunnel: w1415 -> [w1477 w1478]
            tunnel: w1414 -> [w1476 w1479]
            tunnel: [w1477 w1481] -> w1409
            tunnel: [w1476 w1480] -> w1410
            frame False {
            }
            frame True {
              w1483 = 3
              n449 = call "NCS_GetFlowRateMax.vi"("error in (no error)"=w1479, "dosingunit"=w1483, "device handle in"=w1478) -> ("error out"=w1484:errorcluster, "flow rate max"=w1482:dbl, "device handle out"=w1485:u32)
              n450 = call "NCS_EmptySyrige.vi"("error in (no error)"=w1484, "flowrate"=w1482, "dosingunit"=w1483, "device handle in"=w1485) -> ("error out"=w1480:errorcluster, "device handle out"=w1481:u32)
            }
          }
          n451 = case shown="False" "Refill 2" {
            tunnel: w1405 -> [w1457 w1461]
            tunnel: w1406 -> [w1456 w1459]
            tunnel: [w1457 w1460] -> w1401
            tunnel: [w1456 w1458] -> w1398
            frame False {
            }
            frame True {
              w1463 = 1
              n452 = call "NCS_GetFlowRateMax.vi"("error in (no error)"=w1459, "dosingunit"=w1463, "device handle in"=w1461) -> ("error out"=w1464:errorcluster, "flow rate max"=w1462:dbl, "device handle out"=w1465:u32)
              n453 = call "NCS_RefillSyrige.vi"("error in (no error)"=w1464, "flowrate"=w1462, "dosingunit"=w1463, "device handle in"=w1465) -> ("error out"=w1458:errorcluster, "device handle out"=w1460:u32)
            }
          }
          n454 = case shown="False" "Refill 1" {
            tunnel: w1403 -> [w1467 w1475]
            tunnel: w1404 -> [w1466 w1472]
            tunnel: [w1467 w1473] -> w1402
            tunnel: [w1466 w1470] -> w1392
            frame False {
            }
            frame True {
              w1469 = 0
              n455 = call "NCS_GetFlowRateMax.vi"("error in (no error)"=w1472, "dosingunit"=w1469, "device handle in"=w1475) -> ("error out"=w1471:errorcluster, "flow rate max"=w1468:dbl, "device handle out"=w1474:u32)
              n456 = call "NCS_RefillSyrige.vi"("error in (no error)"=w1471, "flowrate"=w1468, "dosingunit"=w1469, "device handle in"=w1474) -> ("error out"=w1470:errorcluster, "device handle out"=w1473:u32)
            }
          }
          n457 = case shown="False" "Refill 3" {
            tunnel: w1407 -> [w1447 w1448]
            tunnel: w1408 -> [w1446 w1449]
            tunnel: [w1447 w1450] -> w1400
            tunnel: [w1446 w1451] -> w1397
            frame False {
            }
            frame True {
              w1453 = 2
              n458 = call "NCS_GetFlowRateMax.vi"("error in (no error)"=w1449, "dosingunit"=w1453, "device handle in"=w1448) -> ("error out"=w1454:errorcluster, "flow rate max"=w1452:dbl, "device handle out"=w1455:u32)
              n459 = call "NCS_RefillSyrige.vi"("error in (no error)"=w1454, "flowrate"=w1452, "dosingunit"=w1453, "device handle in"=w1455) -> ("error out"=w1451:errorcluster, "device handle out"=w1450:u32)
            }
          }
          n460 = case shown="False" "Refill 4" {
            tunnel: w1409 -> [w1437 w1438]
            tunnel: w1410 -> [w1436 w1439]
            tunnel: [w1437 w1441] -> w1399
            tunnel: [w1436 w1440] -> w1396
            frame False {
            }
            frame True {
              w1443 = 3
              n461 = call "NCS_GetFlowRateMax.vi"("error in (no error)"=w1439, "dosingunit"=w1443, "device handle in"=w1438) -> ("error out"=w1444:errorcluster, "flow rate max"=w1442:dbl, "device handle out"=w1445:u32)
              n462 = call "NCS_RefillSyrige.vi"("error in (no error)"=w1444, "flowrate"=w1442, "dosingunit"=w1443, "device handle in"=w1445) -> ("error out"=w1440:errorcluster, "device handle out"=w1441:u32)
            }
          }
        }
      }
      n463 = Or(x=w870, y=w868) -> (x .or. y?=w966:bool)
      n464 = Or(x=w966, y=w869) -> (x .or. y?=w882:bool)
      n465 = Multiply(x="Minutes between Exp", y=60) -> (x*y=w955:dbl)
      n466 = Divide(x=w955, y=5) -> (x/y=w956:dbl)
      n467 = Greater Or Equal?(x=w958, y=w956) -> (x >= y?=w992:bool)
      n468 = Or(x=w992, y=w882) -> (x .or. y?=w978:bool)
      n469 = Or(x=w882, y="Stop everything") -> (x .or. y?=w883:bool)
      n470 = Or(x=w888, y=w883) -> (x .or. y?=w889:bool)
      n471 = case shown="False" w889 {
        tunnel: [w1304 w1379] -> w880
        tunnel: [w1303 w1379] -> w879
        tunnel: [w1302 w1379] -> w878
        tunnel: [w1301 w1379] -> w877
        frame False {
          w1305 = "?BSI_ReadData"  # ?BSI_ReadData
          n472 = stacked-sequence {
            seq-local: [w1306 _ _] -> [_ _ w1362]
            tunnel: w1305 -> [w1306 _ _]
            tunnel: [_ _ w1339] -> w1304
            tunnel: [_ _ w1338] -> w1303
            tunnel: [_ _ w1337] -> w1302
            tunnel: [_ _ w1336] -> w1301
            frame #0 {
              # "Write Text to Clipboard"
              n473 = String Length(string=w1306) -> (length=w1315:i32)
              n474 = Increment(x=w1315) -> (x+1=w1311:i32)
              n475 = dll-call lib="kernel32" fn="GlobalAlloc"("Flags"=i16 0 ("Format"), "Size"=w1311) -> (w1310:i32)  [unwired: 5 in, 2 out]
              n476 = dll-call lib="kernel32" fn="GlobalLock"("hGlobalMemory"=w1310) -> (w1313:i32)  [unwired: 4 in, 2 out]
              n477 = dll-call lib="kernel32" fn="lstrcpy"("Flags"=w1313, "String"=w1306) -> (w1312:i32)  [unwired: 5 in, 2 out]
              n478 = stacked-sequence {
                tunnel: w1312 -> [_]
                tunnel: w1310 -> [w1334]
                tunnel: [w1333] -> w1309
                frame #0 {
                  n479 = dll-call lib="kernel32" fn="LocalUnlock"("hGlobalMemory"=w1334) -> (w1333:i32)  [unwired: 4 in, 2 out]
                }
              }
              "Error Out 2" <- w1309
              n480 = case shown="0" w1309 {
                selector: w1309 -> [_ w1330]
                tunnel: w1310 -> [w1316 _]
                tunnel: [w1317 w1329] -> w1308
                frame 0 {
                  n481 = dll-call lib="user32" fn="OpenClipboard"("owner"=i16 0) -> (w1318:i32)  [unwired: 4 in, 2 out]
                  n482 = case shown="1, Default" w1318 {
                    selector: w1318 -> [w1322 _]
                    tunnel: [w1320 w1325] -> w1317
                    tunnel: w1316 -> [_ w1324]
                    frame 0 {
                      n483 = Equal To 0?(x=w1322) -> (x = 0?=w1323:bool)
                      n484 = Bundle(w1323, w1322, "source"="Error opening clipboard") -> (w1320:cluster{bool, i32, "source":string})  [unwired: 1 in]
                    }
                    frame 1, Default {
                      n485 = stacked-sequence {
                        tunnel: [_ _ _ cluster{bool, i32, "source":string} {FALSE, 0, "source"=""} ("Output Element")] -> w1325
                        tunnel: w1324 -> [_ w1326 _ _]
                        frame #0 {
                          n486 = dll-call lib="user32" fn="EmptyClipboard"() -> ()  [unwired: 4 in, 2 out]
                        }
                        frame #1 {
                          n487 = dll-call lib="user32" fn="SetClipboardData"("Format"=1, "Data"=w1326) -> ()  [unwired: 6 in, 2 out]
                        }
                        frame #2 {
                          n488 = dll-call lib="user32" fn="CloseClipboard"() -> ()  [unwired: 4 in, 2 out]
                        }
                        frame #3 {
                        }
                      }
                    }
                  }
                }
                frame 1, Default {
                  n489 = Not Equal To 0?(x=w1330) -> (x != 0?=w1331:bool)
                  n490 = Bundle(w1331, w1330, "source"="Error copying text to clipboard") -> (w1329:cluster{bool, i32, "source":string})  [unwired: 1 in]
                }
              }
              "Write error out 2" <- w1308
              n491 = local write "Read Flow Status"("Running" ("Status")) -> ()
            }
            frame #1 {
              # "Wait 500 milliseconds"
              n492 = Wait (ms)(milliseconds to wait=u32 500) -> ()  [unwired: 1 out]
            }
            frame #2 {
              # "Read Text From Clipboard"
              n493 = dll-call lib="user32" fn="OpenClipboard"("owner"=i16 0) -> (w1364:i32)  [unwired: 4 in, 2 out]
              n494 = case shown="1, Default" w1364 {
                selector: w1364 -> [w1370 _]
                tunnel: ["" w1375] -> w1354
                tunnel: [w1368 cluster{bool, i32, "source":string} {FALSE, 0, "source"=""} ("Output Element")] -> w1363
                frame 0 {
                  n495 = Equal To 0?(x=w1370) -> (x = 0?=w1371:bool)
                  n496 = Bundle(w1371, w1370, "source"="No text in clipboard available!") -> (w1368:cluster{bool, i32, "source":string})  [unwired: 1 in]
                }
                frame 1, Default {
                  n497 = dll-call lib="user32" fn="GetClipboardData"("uFormat"=1 ("hGlobalMemory")) -> (w1376:i32)  [unwired: 4 in, 2 out]
                  n498 = dll-call lib="kernel32" fn="GlobalLock"("hGlobalMemory"=w1376) -> (w1375:string, "hGlobalMemory"=w1373:i32)  [unwired: 3 in, 2 out]
                  n499 = stacked-sequence {
                    tunnel: w1373 -> [w1378 _]
                    frame #0 {
                      n500 = dll-call lib="kernel32" fn="LocalUnlock"("hGlobalMemory"=w1378) -> ()  [unwired: 5 in, 2 out]
                    }
                    frame #1 {
                      n501 = dll-call lib="user32" fn="CloseClipboard"() -> ()  [unwired: 4 in, 2 out]
                    }
                  }
                }
              }
              "Text Read From Clipboard 2" <- w1354
              "Read error out 2" <- w1363
              n502 = Search/Split String(string=w1354, search string/char (-)=" ") -> (substring before match=→"First waste string":string, match + rest of string=w1356:string)  [unwired: 1 in, 1 out]
              "Rest of string 1" <- w1356
              n503 = Search/Split String(string=w1356, search string/char (-)=",") -> (substring before match=w1351:string, match + rest of string=w1352:string)  [unwired: 1 in, 1 out]
              "First Number" <- w1351
              "Rest of string 2" <- w1352
              n504 = Search/Split String(string=w1352, search string/char (-)="n") -> (substring before match=w1349:string, match + rest of string=w1342:string)  [unwired: 1 in, 1 out]
              "Second Number 2" <- w1349
              "Rest of string 3" <- w1342
              n505 = Search/Split String(string=w1342, search string/char (-)="i") -> (substring before match=w1340:string, match + rest of string=w1345:string)  [unwired: 1 in, 1 out]
              "Third Number 3" <- w1340
              "Rest of string 4" <- w1345
              n506 = Equal?(x=w1362, y=w1354) -> (x = y?=w1361:bool)
              n507 = Search/Split String(string=w1345, search string/char (-)="l") -> (substring before match=w1343:string, match + rest of string=→"Rest of string 5":string)  [unwired: 1 in, 1 out]
              "Fourth Number 3" <- w1343
              n508 = case shown="True" w1361 {
                tunnel: ["Response OK" "Failed: No Response from Lab Interface"] -> w1360
                frame False {
                }
                frame True {
                }
              }
              "Read Flow Status" <- w1360
              n509 = Scan From String(input string=w1351) -> (output 1=w1339:dbl)  [unwired: 4 in, 3 out]
              "Gas Flow 1 NmL/min" <- w1339
              n510 = Scan From String(input string=w1349, initial scan location=1) -> (output 1=w1338:dbl)  [unwired: 3 in, 3 out]
              "Gas Flow 2 NmL/min" <- w1338
              n511 = Scan From String(input string=w1340, initial scan location=2) -> (output 1=w1337:dbl)  [unwired: 3 in, 3 out]
              "Gas Flow 3 NmL/min" <- w1337
              n512 = Scan From String(input string=w1343, initial scan location=3) -> (output 1=w1336:dbl)  [unwired: 3 in, 3 out]
              "Gas Flow 4 NmL/min" <- w1336
              n513 = Merge Signals(w1339, w1338, w1337, w1336) -> (→"Gas Flow rate":dynamicdata)
            }
          }
        }
        frame True {
          w1379 = 0
        }
      }
      n514 = Merge Signals(w948, w947, w925, w950, w977, w976, w903, w902, w901, w900, w880, w879, w878, w877) -> (w996:dynamicdata)
      n515 = call "Write To Measurement File"("Signals"=w996) -> ()  [unwired: 16 in, 3 out]
      n516 = case shown="True" w883 {
        frame False {
        }
        frame True {
          w1056 = "?BSI_SetFlowSetPoints 0,0,0,0,*,*,*,*,*,*,*,*,*,*,*,*,*,*,*,*,*,*,*,*,*,*,*,*,*,*"  # ?BSI_SetFlowSetPoints 0,0,0,0,*,*,*,*,*,*,*,*,*,*,*,*,*,*,*,*,*,*,*,*,*,*,*,*,*,*
          n517 = stacked-sequence {
            seq-local: [w1057 _ _] -> [_ _ w1090]
            tunnel: w1056 -> [w1057 _ _]
            frame #0 {
              # "Write Text to Clipboard"
              n518 = String Length(string=w1057) -> (length=w1066:i32)
              n519 = Increment(x=w1066) -> (x+1=w1062:i32)
              n520 = dll-call lib="kernel32" fn="GlobalAlloc"("Flags"=i16 0 ("Format"), "Size"=w1062) -> (w1061:i32)  [unwired: 5 in, 2 out]
              n521 = dll-call lib="kernel32" fn="GlobalLock"("hGlobalMemory"=w1061) -> (w1064:i32)  [unwired: 4 in, 2 out]
              n522 = dll-call lib="kernel32" fn="lstrcpy"("Flags"=w1064, "String"=w1057) -> (w1063:i32)  [unwired: 5 in, 2 out]
              n523 = stacked-sequence {
                tunnel: w1063 -> [_]
                tunnel: w1061 -> [w1085]
                tunnel: [w1084] -> w1060
                frame #0 {
                  n524 = dll-call lib="kernel32" fn="LocalUnlock"("hGlobalMemory"=w1085) -> (w1084:i32)  [unwired: 4 in, 2 out]
                }
              }
              "Error Out 5" <- w1060
              n525 = case shown="0" w1060 {
                selector: w1060 -> [_ w1081]
                tunnel: w1061 -> [w1067 _]
                tunnel: [w1068 w1080] -> w1059
                frame 0 {
                  n526 = dll-call lib="user32" fn="OpenClipboard"("owner"=i16 0) -> (w1069:i32)  [unwired: 4 in, 2 out]
                  n527 = case shown="1, Default" w1069 {
                    selector: w1069 -> [w1073 _]
                    tunnel: [w1071 w1076] -> w1068
                    tunnel: w1067 -> [_ w1075]
                    tunnel: w1067 -> [_ _]
                    frame 0 {
                      n528 = Equal To 0?(x=w1073) -> (x = 0?=w1074:bool)
                      n529 = Bundle(w1074, w1073, "source"="Error opening clipboard") -> (w1071:cluster{bool, i32, "source":string})  [unwired: 1 in]
                    }
                    frame 1, Default {
                      n530 = stacked-sequence {
                        tunnel: [_ _ _ cluster{bool, i32, "source":string} {FALSE, 0, "source"=""} ("Output Element")] -> w1076
                        tunnel: w1075 -> [_ w1077 _ _]
                        frame #0 {
                          n531 = dll-call lib="user32" fn="EmptyClipboard"() -> ()  [unwired: 4 in, 2 out]
                        }
                        frame #1 {
                          n532 = dll-call lib="user32" fn="SetClipboardData"("Format"=1, "Data"=w1077) -> ()  [unwired: 6 in, 2 out]
                        }
                        frame #2 {
                          n533 = dll-call lib="user32" fn="CloseClipboard"() -> ()  [unwired: 4 in, 2 out]
                        }
                        frame #3 {
                        }
                      }
                    }
                  }
                }
                frame 1, Default {
                  n534 = Not Equal To 0?(x=w1081) -> (x != 0?=w1082:bool)
                  n535 = Bundle(w1082, w1081, "source"="Error copying text to clipboard") -> (w1080:cluster{bool, i32, "source":string})  [unwired: 1 in]
                }
              }
              "Write error out 5" <- w1059
              n536 = local write "Write Set Point Status 2"("Running" ("Status")) -> ()
            }
            frame #1 {
              # "Wait 500 milliseconds"
              n537 = Wait (ms)(milliseconds to wait=u32 500) -> ()  [unwired: 1 out]
            }
            frame #2 {
              # "Read Text From Clipboard"
              n538 = dll-call lib="user32" fn="OpenClipboard"("owner"=i16 0) -> (w1092:i32)  [unwired: 4 in, 2 out]
              n539 = case shown="1, Default" w1092 {
                selector: w1092 -> [w1098 _]
                tunnel: ["" w1103] -> w1087
                tunnel: [w1096 cluster{bool, i32, "source":string} {FALSE, 0, "source"=""} ("Output Element")] -> w1091
                frame 0 {
                  n540 = Equal To 0?(x=w1098) -> (x = 0?=w1099:bool)
                  n541 = Bundle(w1099, w1098, "source"="No text in clipboard available!") -> (w1096:cluster{bool, i32, "source":string})  [unwired: 1 in]
                }
                frame 1, Default {
                  n542 = dll-call lib="user32" fn="GetClipboardData"("uFormat"=1 ("hGlobalMemory")) -> (w1104:i32)  [unwired: 4 in, 2 out]
                  n543 = dll-call lib="kernel32" fn="GlobalLock"("hGlobalMemory"=w1104) -> (w1103:string, "hGlobalMemory"=w1101:i32)  [unwired: 3 in, 2 out]
                  n544 = stacked-sequence {
                    tunnel: w1101 -> [w1106 _]
                    frame #0 {
                      n545 = dll-call lib="kernel32" fn="LocalUnlock"("hGlobalMemory"=w1106) -> ()  [unwired: 5 in, 2 out]
                    }
                    frame #1 {
                      n546 = dll-call lib="user32" fn="CloseClipboard"() -> ()  [unwired: 4 in, 2 out]
                    }
                  }
                }
              }
              "Text Read From Clipboard 5" <- w1087
              "Read error out 5" <- w1091
              n547 = Equal?(x=w1090, y=w1087) -> (x = y?=w1089:bool)
              n548 = case shown="True" w1089 {
                tunnel: ["Response OK" "Failed: No Response from Lab Interface"] -> w1088
                frame False {
                }
                frame True {
                }
              }
              "Write Set Point Status 2" <- w1088
            }
          }
        }
      }
      n549 = Or(x="Skip Exp", y=w978) -> (x .or. y?=w993:bool)
      n550 = Or(x="Stop everything", y=w993) -> (x .or. y?=w884:bool)
      n551 = node-c288() -> ()  [unwired: 1 in, 1 out]
      n552 = Build Array(w1006, w1005, w1004, w1003) -> (w998:u32[])
      n553 = Build Array(w999, w1002, w1001, w1000) -> (w997:errorcluster[])
      "loop ind" <- w958
      "Safety Shut Down Pressure (barg)" <- w904
      "High Conc" <- w923
      "Low Conc" <- w924
    }
    n554 = Or(x=w147, y=w155) -> (x .or. y?=w148:bool)
    n555 = node-c288(w161) -> ()  [unwired: 1 out]
  }
  n556 = call <vilib>:"DAQmx Stop Task.vi"("task/channels in"=w50, "error in"=w49) -> ("task out"=w52:refnum<k21>, "error out"=w51:errorcluster)  [unwired: 12 in]
  n557 = Index Array(array=w75, index=0) -> (element=w77:u32)
  n558 = Index Array(array=w74, index=0) -> (element=w76:errorcluster)
  n559 = call <vilib>:"DAQmx Stop Task.vi"("task/channels in"=w40, "error in"=w38) -> ("task out"=w39:refnum<k21>, "error out"=w41:errorcluster)  [unwired: 12 in]
  n560 = call <vilib>:"DAQmx Clear Task.vi"("task in"=w52, "error in"=w51) -> ()  [unwired: 13 in, 1 out]
  n561 = call <vilib>:"DAQmx Clear Task.vi"("task in"=w39, "error in"=w41) -> ()  [unwired: 13 in, 1 out]
  n562 = call "NCS_CloseDevice.vi"("error in (no error)"=w76, "device handle"=w77) -> ()  [unwired: 1 out]
  n563 = call "CN7500_Write Set Point Value.vi"("Target Set Point Value"=25, "error in (no error)"=w63, "Controller Number"=w66, "VISA In"=w62) -> ("error out"=w68:errorcluster, "VISA Out"=w69:refnum<visa-resource-name>)  [unwired: 6 in]
  n564 = call "CN7500_Close.vi"("error in (no error)"=w68, "VISA resource name"=w69) -> ()  [unwired: 9 in, 1 out]
